vi "projekatSortiranje.vi"() -> ()   [LabVIEW 2014]
uses:
  Timer 2013/Control Timer.ctl
  Timer za drugi sprat/Control Timer2.ctl
  Timer za treci sprat/Control Timer3.ctl
  <vilib>/functionblocks/Edge Detection/Edge Detect/Edge Detect.vi
  <vilib>/functionblocks/FB Core/FB Core.xnode
  <vilib>/functionblocks/NI_FunctionBlock Libraries.lvlib
panel:
  in  "Kontrola sistema":T1(tab)
  out "Trenutno stanje":T2(ring)
  out "Trenutni paket":enum16{"Nema paketa", "P1", "P2", "P3"}(ring)
  out "Sledeci paket":enum16{"Nema paketa", "P1", "P2", "P3"}(ring)
  out "Sacuvano stanje":T2(ring)
  out "Status prvog tajmera":cluster{"Running":bool, "Done":bool}
  out "Status drugog tajmera":cluster{"Running":bool, "Done":bool}
  out "Status treceg tajmera":cluster{"Running":bool, "Done":bool}
  out "Stop":bool
  out "Emergency Stop":bool
  out "Timer Data Out za prvi sprat":T3
  out "Stanje tajmera 1 - sacuvano":enum16{"Running", "Waiting"}(ring)
  out "Stanja tajmera za sprat 1":enum16{"Running", "Waiting"}(ring)
  out "Timer Data Out za drugi sprat":T3
  out "Stanja tajmera za sprat 2":enum16{"Running", "Waiting"}(ring)
  out "Stanja tajmera 2 - sacuvano":enum16{"Running", "Waiting"}(ring)
  out "Timer Data Out za treci sprat":T3
  out "Stanja tajmera 3 - sacuvano":enum16{"Running", "Waiting"}(ring)
  out "Stanja tajmera za sprat 3":enum16{"Running", "Waiting"}(ring)
  out "Vreme 1":dbl
  out "Vreme 2":dbl
  out "Vreme 3":dbl
  in  "error in":errorcluster
  out "error out":errorcluster
  out "DO0":bool
  out "DO1":bool
  out "DO2":bool
  out "DO3":bool
  out "DO4":bool
  out "DO5":bool
  out "DO6":bool
  out "DO7":bool
  out "DO8":bool
  out "DO9":bool
  out "DO10":bool
  out "DO11":bool
  out "DO12":bool
  out "DO15":bool
  out "DO14":bool
  out "DO13":bool
  in  "Paketi":enum16{"Nema paketa", "P1", "P2", "P3"}(ring)
  in  "Stanja":T2(ring)
  in  "Stanja za odredjivanje paketa":enum16{"B2", "B4", "P3", "P2", "P1", "B3"}(ring)
  in  "Stanja tajmera za spratove":enum16{"Running", "Waiting"}(ring)
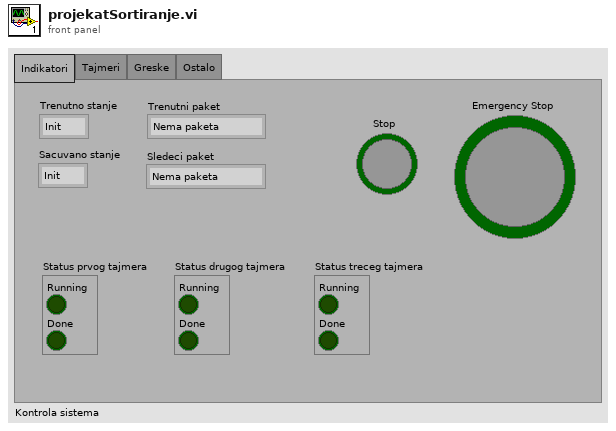
[diagram p1: front panel]
types:
  T1 = enum32{"Indikatori", "Tajmeri", "Greske", "Ostalo"}
  T2 = enum16{"Init", "Wait", "P1", "P2", "P3", "Sledeci paket", "K1", "K7", "K6", "K5", "K4", "K3", "K2", "Emergency Shutdown", "Shutdown"}
  T3 = cluster{"Last Time Stamp":dbl, "Elapsed Time":dbl}
  T4 = typedef "Control Timer3.ctl" = enum16{"Timecheck", "Reset"}
  T5 = typedef "Control Timer2.ctl" = enum16{"Timecheck", "Reset"}
  T6 = typedef "Control Timer.ctl" = enum16{"Timecheck", "Reset"}
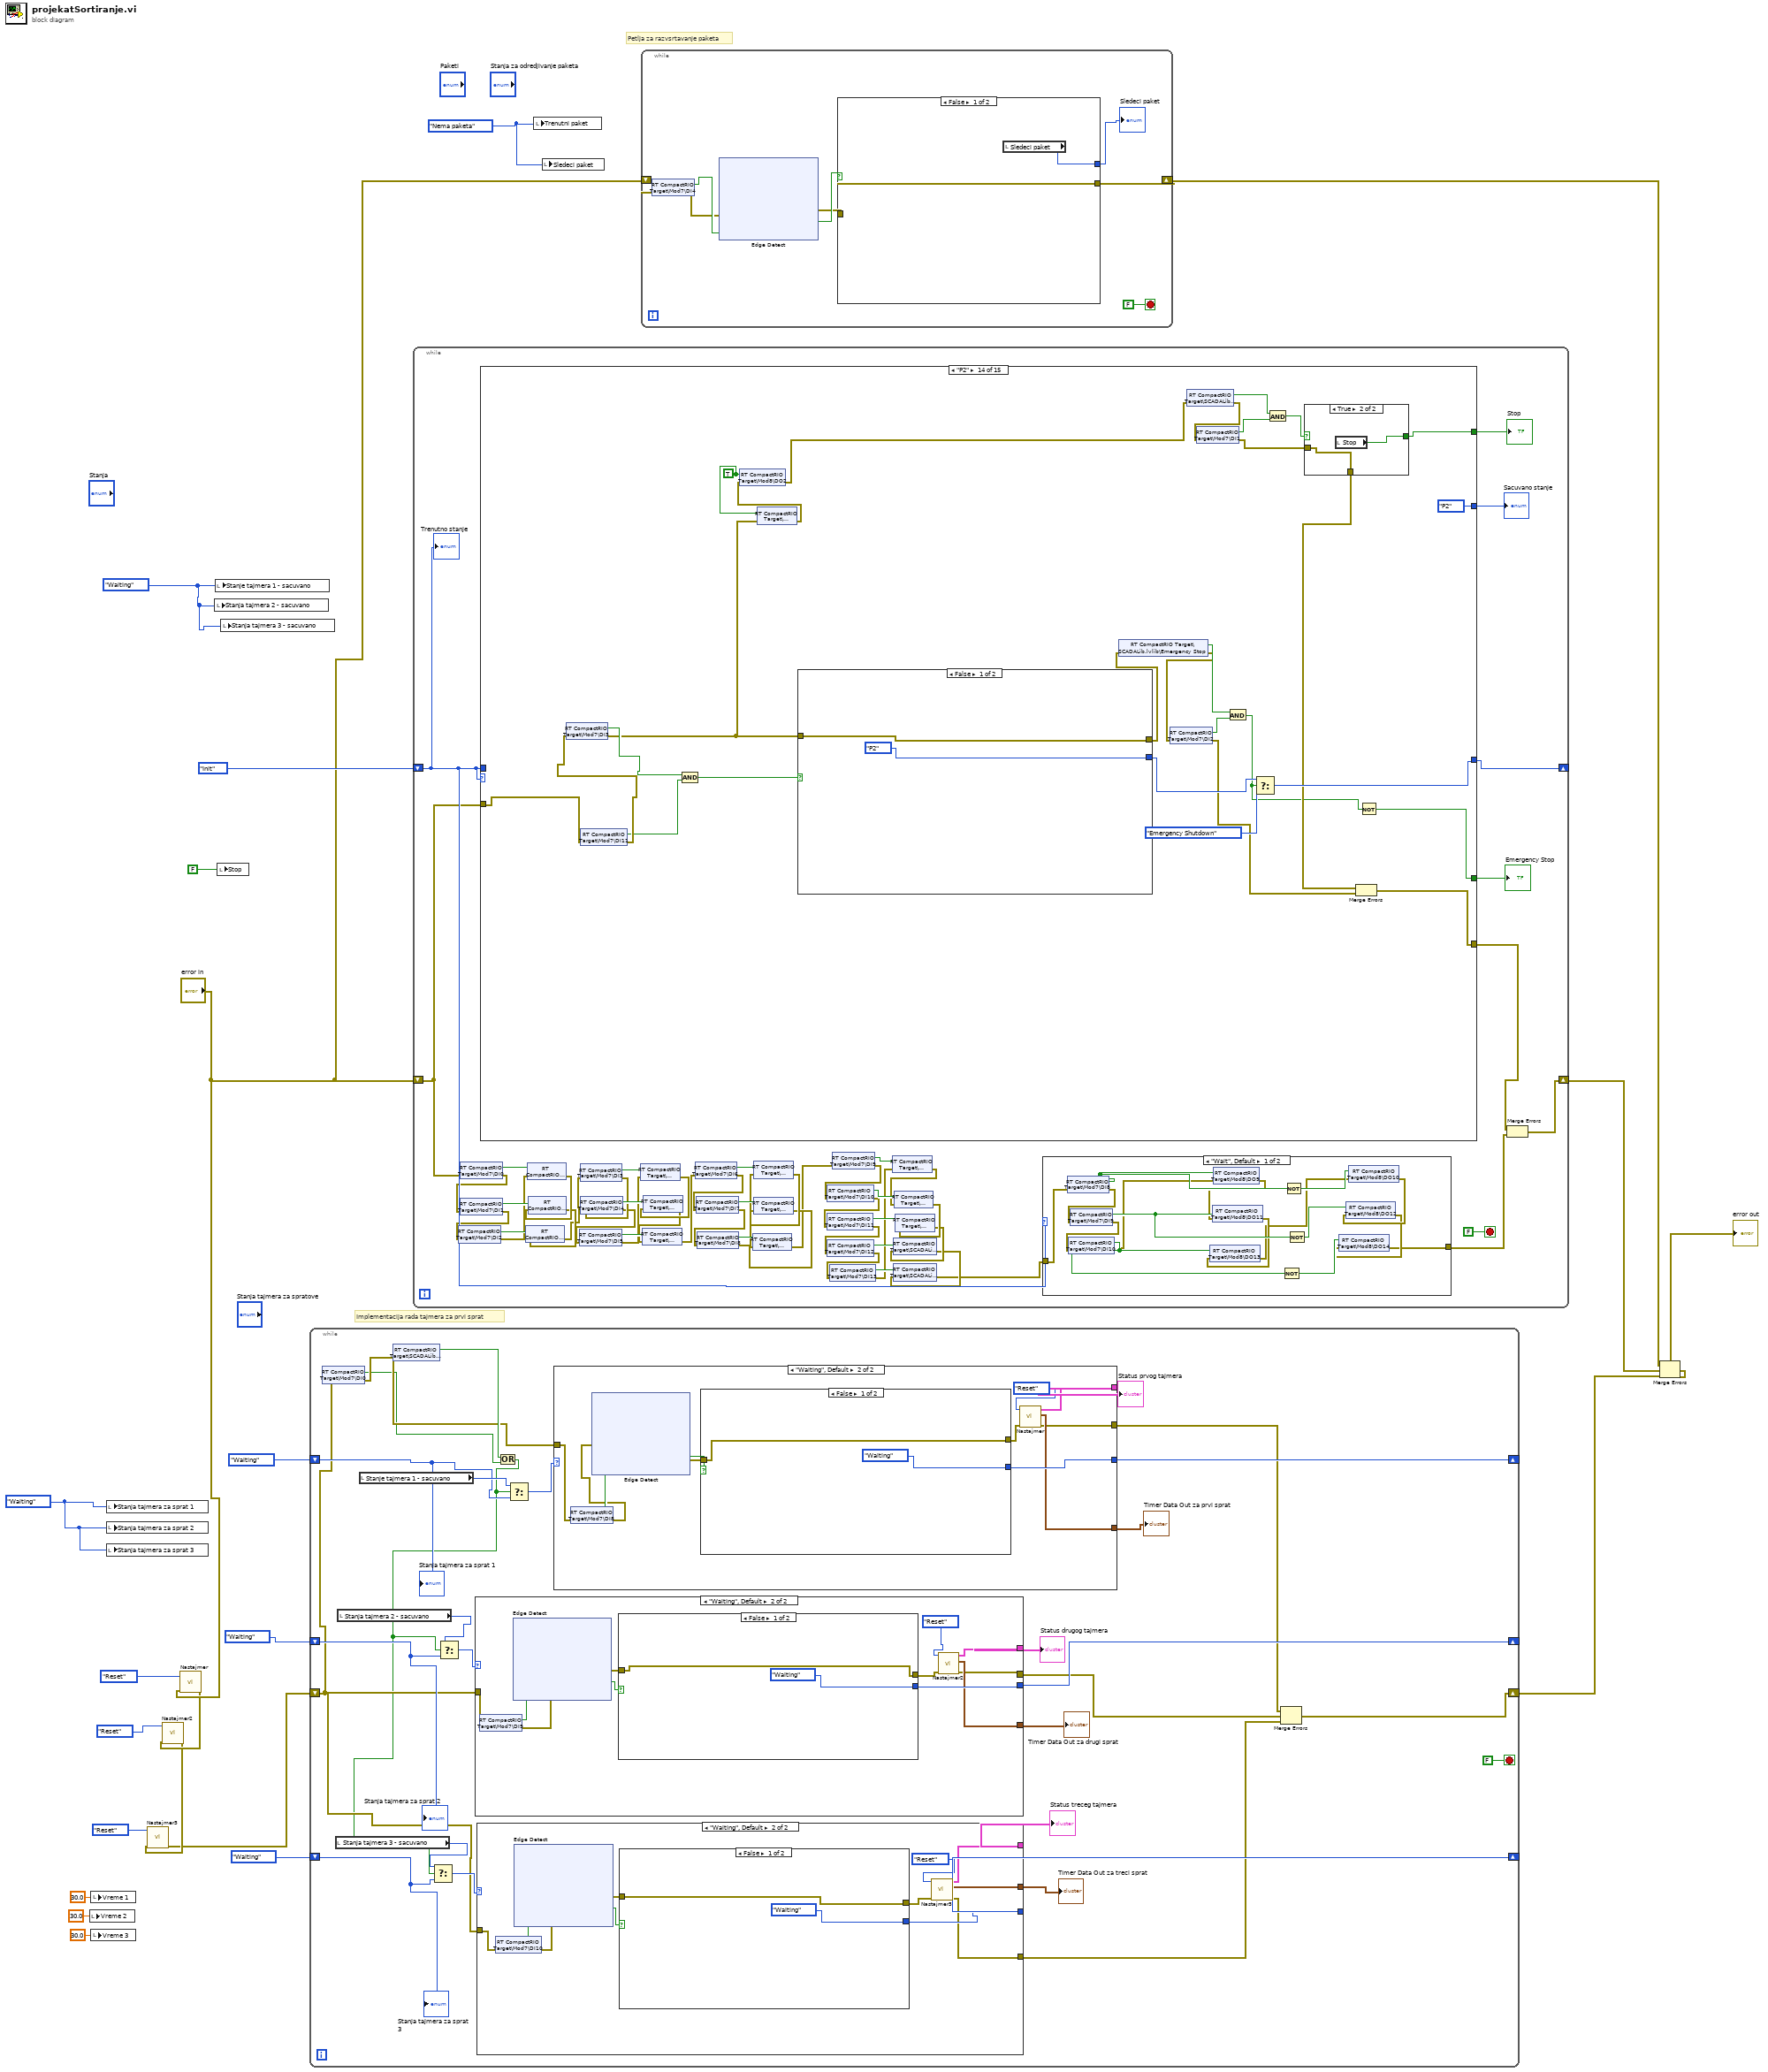
[diagram p0: block diagram]
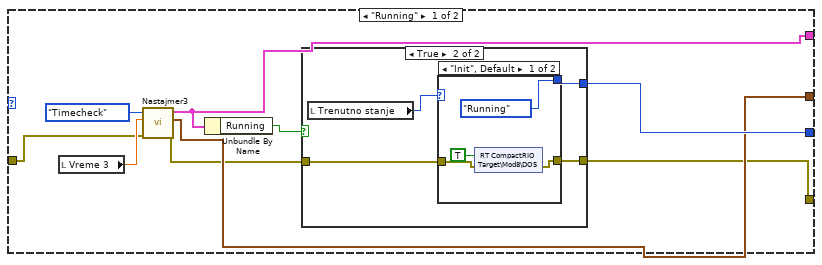
[diagram p2: hidden frame]
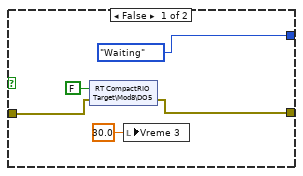
[diagram p3: hidden frame]
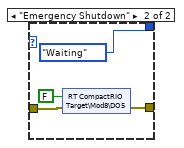
[diagram p4: hidden frame]
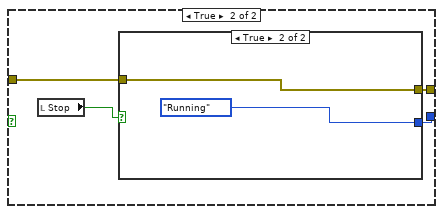
[diagram p5: hidden frame]
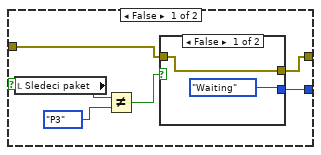
[diagram p6: hidden frame]
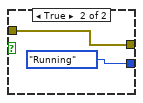
[diagram p7: hidden frame]
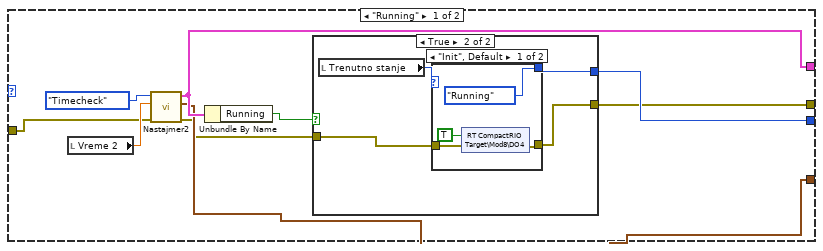
[diagram p8: hidden frame]
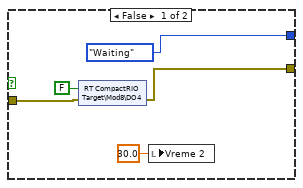
[diagram p9: hidden frame]
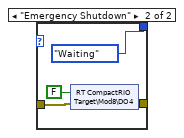
[diagram p10: hidden frame]
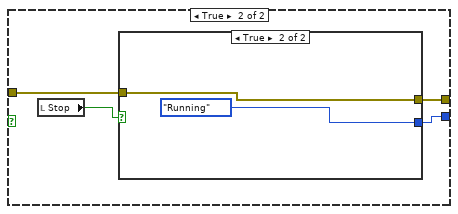
[diagram p11: hidden frame]
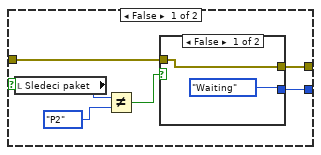
[diagram p12: hidden frame]
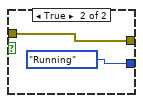
[diagram p13: hidden frame]
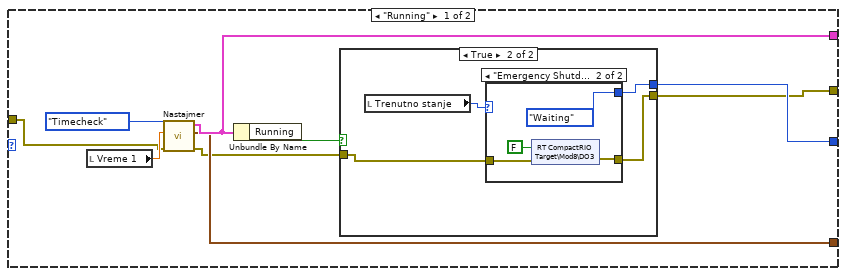
[diagram p14: hidden frame]
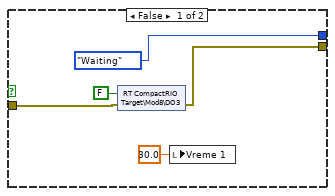
[diagram p15: hidden frame]
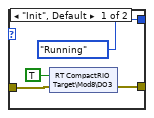
[diagram p16: hidden frame]
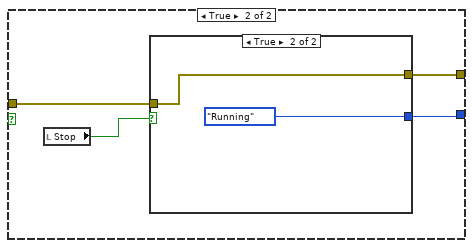
[diagram p17: hidden frame]
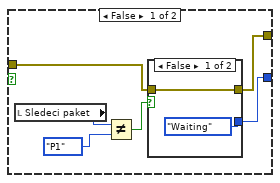
[diagram p18: hidden frame]
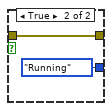
[diagram p19: hidden frame]
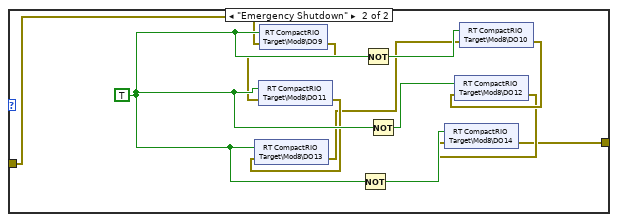
[diagram p20: hidden frame]
diagram:
  w12 = enum16{"Running", "Waiting"}."Waiting" ("Stanja tajmera za sprat 1 - sacuvano")
  w17 = enum16{"Running", "Waiting"}."Waiting" ("Stanja tajmera za spratove 1")
  w18 = enum16{"Nema paketa", "P1", "P2", "P3"}."Nema paketa" ("Trenutni paket")
  # "Implementacija rada tajmera za prvi sprat"
  # "Petlja za razvsrtavanje paketa"
  n1 = local write "Vreme 2"(30.0 ("Vreme 1")) -> ()
  n2 = local write "Vreme 1"(30.0 ("Vreme 1")) -> ()
  n3 = local write "Vreme 3"(30.0 ("Vreme 1")) -> ()
  n4 = local write "Stanja tajmera za sprat 1"(w17) -> ()
  n5 = local write "Stanja tajmera za sprat 2"(w17) -> ()
  n6 = local write "Stanja tajmera za sprat 3"(w17) -> ()
  n7 = call "Nastajmer.vi"("error in (no error)"="error in", "Enum"=Control_Timer."Reset") -> ("error out"=w4:errorcluster)  [unwired: 7 in, 2 out]
  n8 = call "Nastajmer2.vi"("error in (no error)"=w4, "Enum"=Control_Timer2."Reset") -> ("error out"=w3:errorcluster)  [unwired: 7 in, 2 out]
  n9 = call "Nastajmer3.vi"("error in (no error)"=w3, "Enum"=Control_Timer3."Reset") -> ("error out"=w2:errorcluster)  [unwired: 7 in, 2 out]
  n10 = local write "Stanja tajmera 2 - sacuvano"(w12) -> ()
  n11 = local write "Stanje tajmera 1 - sacuvano"(w12) -> ()
  n12 = local write "Stop"(FALSE ("System Stop")) -> ()
  n13 = local write "Stanja tajmera 3 - sacuvano"(w12) -> ()
  n14 = while {
    shift-right: [w49] -> _
    shift-left: enum16{"Running", "Waiting"}."Waiting" ("Stanja tajmera za spratove") -> [w40]
    shift-right: [w47] -> _
    shift-left: enum16{"Running", "Waiting"}."Waiting" ("Stanja tajmera za spratove") -> [w37]
    shift-right: [w46] -> _
    shift-left: enum16{"Running", "Waiting"}."Waiting" ("Stanja tajmera za spratove") -> [w34]
    shift-right: [w28] -> w1
    shift-left: w2 -> [w32]
    stop <- FALSE stop-if-true
    n15 = shared-variable "RT CompactRIO Target\\Mod7\\DI0"(error in=w32) -> (w23:bool, error out=w25:errorcluster)
    n16 = local read "Stanja tajmera 3 - sacuvano"() -> (w35:enum16{"Running", "Waiting"})
    n17 = local read "Stanja tajmera 2 - sacuvano"() -> (w38:enum16{"Running", "Waiting"})
    n18 = local read "Stanje tajmera 1 - sacuvano"() -> (w41:enum16{"Running", "Waiting"})
    n19 = shared-variable "RT CompactRIO Target\\SCADALib.lvlib\\Start"(error in=w25) -> (w26:bool, error out=w24:errorcluster)
    n20 = Or(x=w26, y=w23) -> (x .or. y?=w27:bool)
    n21 = Select(t=w35, s=w27, f=w34) -> (s? t:f=w33:enum16{"Running", "Waiting"})
    n22 = Select(t=w38, s=w27, f=w37) -> (s? t:f=w36:enum16{"Running", "Waiting"})
    n23 = case shown="\"Waiting\", Default" w36 {
      tunnel: [w155 w181] -> w47
      tunnel: [w153 w179] -> w48
      tunnel: [w152 w178] -> w43
      tunnel: w32 -> [w149 w177]
      tunnel: [w147 w173] -> w30
      frame "Running" {
        n24 = local read "Vreme 2"() -> (w150:dbl)
        n25 = call "Nastajmer2.vi"("error in (no error)"=w149, "Time Target"=w150, "Enum"=Control_Timer."Timecheck") -> ("error out"=w148:errorcluster, "Timer Data Out"=w152:T3, "Status"=w153:cluster{"Running":bool, "Done":bool})  [unwired: 6 in]
        n26 = Unbundle By Name(w153) -> ("Running"=w151:bool)
        n27 = case shown="True" w151 {
          tunnel: [enum16{"Running", "Waiting"}."Waiting" ("Stanja tajmera za spratove") w164] -> w155
          tunnel: w148 -> [w157 w162]
          tunnel: [w156 w161] -> w147
          frame False {
            n28 = shared-variable "RT CompactRIO Target\\Mod8\\DO4"(FALSE ("DO3"), error in=w157) -> (error out=w156:errorcluster)
            n29 = local write "Vreme 2"(30.0 ("Vreme 1")) -> ()
          }
          frame True {
            n30 = local read "Trenutno stanje"() -> (w163:T2)
            n31 = case shown="\"Init\", Default" w163 {
              tunnel: [enum16{"Running", "Waiting"}."Running" ("Stanja tajmera za spratove") enum16{"Running", "Waiting"}."Waiting" ("Stanja tajmera za spratove")] -> w164
              tunnel: w162 -> [w166 w170]
              tunnel: [w165 w169] -> w161
              frame "Init", Default {
                n32 = shared-variable "RT CompactRIO Target\\Mod8\\DO4"(TRUE ("DO3"), error in=w166) -> (error out=w165:errorcluster)
              }
              frame "Emergency Shutdown" {
                n33 = shared-variable "RT CompactRIO Target\\Mod8\\DO4"(FALSE ("DO3"), error in=w170) -> (error out=w169:errorcluster)
              }
            }
          }
        }
      }
      frame "Waiting", Default {
        n34 = shared-variable "RT CompactRIO Target\\Mod7\\DI9"(error in=w177) -> (w183:bool, error out=w176:errorcluster)
        n35 = xnode "Edge Detect"("error in"=w176, "input 2"=w183) -> ("error out"=w174:errorcluster, "output"=w182:bool)  [unwired: 1 in]
        n36 = case shown="False" w182 {
          tunnel: [enum16{"Running", "Waiting"}."Waiting" ("Stanja tajmera za spratove") w189] -> w181
          tunnel: [w184 w187] -> w175
          tunnel: w174 -> [w184 w186]
          frame False {
          }
          frame True {
            n37 = local read "Stop"() -> (w188:bool)
            n38 = case shown="True" w188 {
              tunnel: [w192 enum16{"Running", "Waiting"}."Running" ("Stanja tajmera za spratove")] -> w189
              tunnel: [w191 w200] -> w187
              tunnel: w186 -> [w190 w200]
              frame False {
                n39 = local read "Sledeci paket"() -> (w194:enum16{"Nema paketa", "P1", "P2", "P3"})
                n40 = Not Equal?(x=w194, y=enum16{"Nema paketa", "P1", "P2", "P3"}."P2" ("Paket")) -> (x != y?=w193:bool)
                n41 = case shown="False" w193 {
                  tunnel: [enum16{"Running", "Waiting"}."Waiting" ("Stanja tajmera za spratove") enum16{"Running", "Waiting"}."Running" ("Stanja tajmera za spratove")] -> w192
                  tunnel: [w196 w198] -> w191
                  tunnel: w190 -> [w196 w198]
                  frame False {
                  }
                  frame True {
                  }
                }
              }
              frame True {
              }
            }
          }
        }
        n42 = call "Nastajmer2.vi"("error in (no error)"=w175, "Enum"=Control_Timer."Reset") -> ("error out"=w173:errorcluster, "Timer Data Out"=w178:T3, "Status"=w179:cluster{"Running":bool, "Done":bool})  [unwired: 7 in]
      }
    }
    "Status drugog tajmera" <- w48
    "Timer Data Out za drugi sprat" <- w43
    n43 = case shown="\"Waiting\", Default" w33 {
      tunnel: [w60 w86] -> w46
      tunnel: [w57 w84] -> w45
      tunnel: [w58 w83] -> w42
      tunnel: w32 -> [w54 w82]
      tunnel: [w52 w78] -> w31
      frame "Running" {
        n44 = local read "Vreme 3"() -> (w55:dbl)
        n45 = call "Nastajmer3.vi"("error in (no error)"=w54, "Time Target"=w55, "Enum"=Control_Timer."Timecheck") -> ("error out"=w53:errorcluster, "Timer Data Out"=w58:T3, "Status"=w57:cluster{"Running":bool, "Done":bool})  [unwired: 6 in]
        n46 = Unbundle By Name(w57) -> ("Running"=w56:bool)
        n47 = case shown="True" w56 {
          tunnel: [enum16{"Running", "Waiting"}."Waiting" ("Stanja tajmera za spratove") w69] -> w60
          tunnel: w53 -> [w62 w67]
          tunnel: [w61 w66] -> w52
          frame False {
            n48 = shared-variable "RT CompactRIO Target\\Mod8\\DO5"(FALSE ("DO3"), error in=w62) -> (error out=w61:errorcluster)
            n49 = local write "Vreme 3"(30.0 ("Vreme 1")) -> ()
          }
          frame True {
            n50 = local read "Trenutno stanje"() -> (w68:T2)
            n51 = case shown="\"Init\", Default" w68 {
              tunnel: [enum16{"Running", "Waiting"}."Running" ("Stanja tajmera za spratove") enum16{"Running", "Waiting"}."Waiting" ("Stanja tajmera za spratove")] -> w69
              tunnel: w67 -> [w71 w75]
              tunnel: [w70 w74] -> w66
              frame "Init", Default {
                n52 = shared-variable "RT CompactRIO Target\\Mod8\\DO5"(TRUE ("DO3"), error in=w71) -> (error out=w70:errorcluster)
              }
              frame "Emergency Shutdown" {
                n53 = shared-variable "RT CompactRIO Target\\Mod8\\DO5"(FALSE ("DO3"), error in=w75) -> (error out=w74:errorcluster)
              }
            }
          }
        }
      }
      frame "Waiting", Default {
        n54 = shared-variable "RT CompactRIO Target\\Mod7\\DI10"(error in=w82) -> (w88:bool, error out=w81:errorcluster)
        n55 = xnode "Edge Detect"("error in"=w81, "input 2"=w88) -> ("error out"=w80:errorcluster, "output"=w87:bool)  [unwired: 1 in]
        n56 = case shown="False" w87 {
          tunnel: [enum16{"Running", "Waiting"}."Waiting" ("Stanja tajmera za spratove") w94] -> w86
          tunnel: [w89 w92] -> w79
          tunnel: w80 -> [w89 w91]
          frame False {
          }
          frame True {
            n57 = local read "Stop"() -> (w93:bool)
            n58 = case shown="True" w93 {
              tunnel: [w97 enum16{"Running", "Waiting"}."Running" ("Stanja tajmera za spratove")] -> w94
              tunnel: [w96 w105] -> w92
              tunnel: w91 -> [w95 w105]
              frame False {
                n59 = local read "Sledeci paket"() -> (w99:enum16{"Nema paketa", "P1", "P2", "P3"})
                n60 = Not Equal?(x=w99, y=enum16{"Nema paketa", "P1", "P2", "P3"}."P3" ("Paket")) -> (x != y?=w98:bool)
                n61 = case shown="False" w98 {
                  tunnel: [enum16{"Running", "Waiting"}."Waiting" ("Stanja tajmera za spratove") enum16{"Running", "Waiting"}."Running" ("Stanja tajmera za spratove")] -> w97
                  tunnel: [w101 w103] -> w96
                  tunnel: w95 -> [w101 w103]
                  frame False {
                  }
                  frame True {
                  }
                }
              }
              frame True {
              }
            }
          }
        }
        n62 = call "Nastajmer3.vi"("error in (no error)"=w79, "Enum"=Control_Timer."Reset") -> ("error out"=w78:errorcluster, "Timer Data Out"=w83:T3, "Status"=w84:cluster{"Running":bool, "Done":bool})  [unwired: 7 in]
      }
    }
    "Status treceg tajmera" <- w45
    "Timer Data Out za treci sprat" <- w42
    n63 = Select(t=w41, s=w27, f=w40) -> (s? t:f=w39:enum16{"Running", "Waiting"})
    n64 = case shown="\"Waiting\", Default" w39 {
      tunnel: [w250 w277] -> w49
      tunnel: [w247 w274] -> w50
      tunnel: [w246 w273] -> w44
      tunnel: w24 -> [w244 w272]
      tunnel: [w242 w268] -> w29
      frame "Running" {
        n65 = local read "Vreme 1"() -> (w245:dbl)
        n66 = call "Nastajmer.vi"("error in (no error)"=w244, "Time Target"=w245, "Enum"=Control_Timer."Timecheck") -> ("error out"=w243:errorcluster, "Timer Data Out"=w246:T3, "Status"=w247:cluster{"Running":bool, "Done":bool})  [unwired: 6 in]
        n67 = Unbundle By Name(w247) -> ("Running"=w248:bool)
        n68 = case shown="True" w248 {
          tunnel: [enum16{"Running", "Waiting"}."Waiting" ("Stanja tajmera za spratove") w259] -> w250
          tunnel: w243 -> [w252 w257]
          tunnel: [w251 w256] -> w242
          frame False {
            n69 = shared-variable "RT CompactRIO Target\\Mod8\\DO3"(FALSE ("DO3"), error in=w252) -> (error out=w251:errorcluster)
            n70 = local write "Vreme 1"(30.0 ("Vreme 1")) -> ()
          }
          frame True {
            n71 = local read "Trenutno stanje"() -> (w258:T2)
            n72 = case shown="\"Emergency Shutdown\"" w258 {
              tunnel: [enum16{"Running", "Waiting"}."Running" ("Stanja tajmera za spratove") enum16{"Running", "Waiting"}."Waiting" ("Stanja tajmera za spratove")] -> w259
              tunnel: w257 -> [w261 w265]
              tunnel: [w260 w264] -> w256
              frame "Init", Default {
                n73 = shared-variable "RT CompactRIO Target\\Mod8\\DO3"(TRUE ("DO3"), error in=w261) -> (error out=w260:errorcluster)
              }
              frame "Emergency Shutdown" {
                n74 = shared-variable "RT CompactRIO Target\\Mod8\\DO3"(FALSE ("DO3"), error in=w265) -> (error out=w264:errorcluster)
              }
            }
          }
        }
      }
      frame "Waiting", Default {
        n75 = shared-variable "RT CompactRIO Target\\Mod7\\DI8"(error in=w272) -> (w278:bool, error out=w271:errorcluster)
        n76 = xnode "Edge Detect"("error in"=w271, "input 2"=w278) -> ("error out"=w269:errorcluster, "output"=w276:bool)  [unwired: 1 in]
        n77 = case shown="False" w276 {
          tunnel: [enum16{"Running", "Waiting"}."Waiting" ("Stanja tajmera za spratove") w283] -> w277
          tunnel: [w279 w282] -> w270
          tunnel: w269 -> [w279 w281]
          frame False {
          }
          frame True {
            n78 = local read "Stop"() -> (w284:bool)
            n79 = case shown="True" w284 {
              tunnel: [w287 enum16{"Running", "Waiting"}."Running" ("Stanja tajmera za spratove")] -> w283
              tunnel: [w286 w295] -> w282
              tunnel: w281 -> [w285 w295]
              frame False {
                n80 = local read "Sledeci paket"() -> (w290:enum16{"Nema paketa", "P1", "P2", "P3"})
                n81 = Not Equal?(x=w290, y=enum16{"Nema paketa", "P1", "P2", "P3"}."P1" ("Paket")) -> (x != y?=w288:bool)
                n82 = case shown="False" w288 {
                  tunnel: [enum16{"Running", "Waiting"}."Waiting" ("Stanja tajmera za spratove") enum16{"Running", "Waiting"}."Running" ("Stanja tajmera za spratove")] -> w287
                  tunnel: [w291 w293] -> w286
                  tunnel: w285 -> [w291 w293]
                  frame False {
                  }
                  frame True {
                  }
                }
              }
              frame True {
              }
            }
          }
        }
        n83 = call "Nastajmer.vi"("error in (no error)"=w270, "Enum"=Control_Timer."Reset") -> ("error out"=w268:errorcluster, "Timer Data Out"=w273:T3, "Status"=w274:cluster{"Running":bool, "Done":bool})  [unwired: 7 in]
      }
    }
    "Status prvog tajmera" <- w50
    "Timer Data Out za prvi sprat" <- w44
    n84 = Merge Errors(w29, w30, w31) -> (w28:errorcluster)
    "Stanja tajmera za sprat 1" <- w40
    "Stanja tajmera za sprat 2" <- w37
    "Stanja tajmera za sprat 3" <- w34
  }
  n85 = while {
    shift-right: [w380] -> w7
    shift-left: "error in" -> [w365]
    shift-right: [w387] -> _
    shift-left: T2."Init" ("Stanja") -> [w383]
    stop <- FALSE stop-if-true
    n86 = shared-variable "RT CompactRIO Target\\Mod7\\DI0"(error in=w365) -> (w379:bool, error out=w364:errorcluster)
    n87 = shared-variable "RT CompactRIO Target\\Mod7\\DI1"(error in=w364) -> (w378:bool, error out=w363:errorcluster)
    n88 = shared-variable "RT CompactRIO Target\\Mod7\\DI2"(error in=w363) -> (w377:bool, error out=w362:errorcluster)
    n89 = case shown="\"P2\"" w383 {
      tunnel: [w416 w467 w506 w545 w631 w791 w860 w957 w990 w1034 w1066 w1229 w1253 w1292 w1331] -> w381
      tunnel: [w446 w474 w505 w566 w633 w788 w859 w968 w1003 w1038 w1073 w1233 w1264 w1303 w1342] -> w387
      tunnel: w383 -> [_ _ _ _ _ _ _ _ _ _ _ w1233 _ _ _]
      tunnel: w365 -> [w418 w453 w482 w550 w629 w800 w851 w965 w1000 w1023 w1054 w1224 w1261 w1300 w1339]
      tunnel: [w447 w473 w501 w562 w618 w803 w847 w961 w996 w1030 w1074 w1232 w1258 w1297 w1336] -> w386
      tunnel: [w444 w470 w498 w559 w616 w802 w845 w959 w994 w1028 w1058 FALSE w1256 w1294 w1334] -> w385
      tunnel: [T2."Init" ("Stanja") T2."Wait" ("Stanja") T2."K1" ("Stanja") T2."Sledeci paket" ("Stanja") T2."K7" ("Stanja") T2."K6" ("Stanja") T2."K5" ("Stanja") T2."K3" ("Stanja") T2."K4" ("Stanja") T2."K2" ("Stanja") w1072 T2."Shutdown" ("Sacuvano stanje") T2."P1" ("Sacuvano stanje") T2."P2" ("Sacuvano stanje") T2."P3" ("Sacuvano stanje")] -> w384
      frame "Init" {
        w434 = FALSE
        n90 = shared-variable "RT CompactRIO Target\\Mod8\\DO0"(w434, error in=w418) -> (error out=w433:errorcluster)
        n91 = shared-variable "RT CompactRIO Target\\Mod8\\DO1"(w434, error in=w433) -> (error out=w432:errorcluster)
        n92 = shared-variable "RT CompactRIO Target\\Mod8\\DO2"(w434, error in=w432) -> (error out=w431:errorcluster)
        n93 = shared-variable "RT CompactRIO Target\\Mod8\\DO3"(w434, error in=w431) -> (error out=w430:errorcluster)
        n94 = shared-variable "RT CompactRIO Target\\Mod8\\DO4"(w434, error in=w430) -> (error out=w429:errorcluster)
        n95 = shared-variable "RT CompactRIO Target\\Mod8\\DO5"(w434, error in=w429) -> (error out=w428:errorcluster)
        n96 = shared-variable "RT CompactRIO Target\\Mod8\\DO6"(w434, error in=w428) -> (error out=w427:errorcluster)
        n97 = shared-variable "RT CompactRIO Target\\Mod8\\DO7"(w434, error in=w427) -> (error out=w424:errorcluster)
        n98 = shared-variable "RT CompactRIO Target\\Mod8\\DO8"(w434, error in=w424) -> (error out=w426:errorcluster)
        n99 = shared-variable "RT CompactRIO Target\\Mod8\\DO9"(w434, error in=w426) -> (error out=w423:errorcluster)
        n100 = shared-variable "RT CompactRIO Target\\Mod8\\DO10"(w434, error in=w423) -> (error out=w425:errorcluster)
        n101 = shared-variable "RT CompactRIO Target\\Mod8\\DO11"(w434, error in=w425) -> (error out=w422:errorcluster)
        n102 = shared-variable "RT CompactRIO Target\\Mod8\\DO12"(w434, error in=w422) -> (error out=w421:errorcluster)
        n103 = shared-variable "RT CompactRIO Target\\Mod8\\DO13"(w434, error in=w421) -> (error out=w420:errorcluster)
        n104 = shared-variable "RT CompactRIO Target\\Mod8\\DO14"(w434, error in=w420) -> (error out=w419:errorcluster)
        n105 = shared-variable "RT CompactRIO Target\\Mod8\\DO15"(w434, error in=w419) -> (error out=w417:errorcluster)
        n106 = shared-variable "RT CompactRIO Target\\SCADALib.lvlib\\Stop"(error in=w417) -> (w439:bool, error out=w441:errorcluster)
        n107 = shared-variable "RT CompactRIO Target\\Mod7\\DI1"(error in=w441) -> (w438:bool, error out=w440:errorcluster)
        n108 = And(x=w439, y=w438) -> (x .and. y?=w442:bool)
        n109 = case shown="True" w442 {
          tunnel: [TRUE w451] -> w447
          tunnel: w440 -> [w448 w450]
          tunnel: [w448 w450] -> w437
          frame False {
          }
          frame True {
            n110 = local read "Stop"() -> (w451:bool)
          }
        }
        n111 = shared-variable "RT CompactRIO Target\\Mod7\\DI2"(error in=w437) -> (w445:bool, error out=w416:errorcluster)
        n112 = Not(x=w445) -> (.not. x?=w444:bool)
        n113 = Select(t=T2."Wait" ("Stanja"), s=w445, f=T2."Emergency Shutdown" ("Stanja")) -> (s? t:f=w446:T2)
      }
      frame "Wait" {
        n114 = shared-variable "RT CompactRIO Target\\SCADALib.lvlib\\Start"(error in=w453) -> (w464:bool, error out=w452:errorcluster)
        n115 = shared-variable "RT CompactRIO Target\\Mod7\\DI0"(error in=w452) -> (w466:bool, error out=w455:errorcluster)
        n116 = Or(x=w466, y=w464) -> (x .or. y?=w465:bool)
        n117 = Select(t=T2."K1" ("Stanja"), s=w465, f=T2."Wait" ("Stanja")) -> (s? t:f=w472:T2)
        n118 = shared-variable "RT CompactRIO Target\\SCADALib.lvlib\\Emergency Stop"(error in=w455) -> (w461:bool, error out=w454:errorcluster)
        n119 = shared-variable "RT CompactRIO Target\\Mod7\\DI2"(error in=w454) -> (w462:bool, error out=w457:errorcluster)
        n120 = And(x=w462, y=w461) -> (x .and. y?=w463:bool)
        n121 = Select(t=w472, s=w463, f=T2."Emergency Shutdown" ("Stanja")) -> (s? t:f=w474:T2)
        n122 = Not(x=w463) -> (.not. x?=w470:bool)
        n123 = shared-variable "RT CompactRIO Target\\SCADALib.lvlib\\Stop"(error in=w457) -> (w458:bool, error out=w456:errorcluster)
        n124 = shared-variable "RT CompactRIO Target\\Mod7\\DI1"(error in=w456) -> (w460:bool, error out=w468:errorcluster)
        n125 = And(x=w458, y=w460) -> (x .and. y?=w459:bool)
        n126 = case shown="True" w459 {
          tunnel: [TRUE w480] -> w473
          tunnel: [w477 w479] -> w467
          tunnel: w468 -> [w477 w479]
          frame False {
          }
          frame True {
            n127 = local read "Stop"() -> (w480:bool)
          }
        }
      }
      frame "K1" {
        w483 = TRUE ("K1")
        n128 = local read "Sledeci paket"() -> (w504:enum16{"Nema paketa", "P1", "P2", "P3"})
        n129 = shared-variable "RT CompactRIO Target\\SCADALib.lvlib\\On-Off"(w483, error in=w482) -> (error out=w481:errorcluster)
        n130 = shared-variable "RT CompactRIO Target\\Mod8\\DO0"(w483, error in=w481) -> (error out=w491:errorcluster)
        n131 = shared-variable "RT CompactRIO Target\\SCADALib.lvlib\\Emergency Stop"(error in=w491) -> (w492:bool, error out=w490:errorcluster)
        n132 = shared-variable "RT CompactRIO Target\\Mod7\\DI2"(error in=w490) -> (w493:bool, error out=w485:errorcluster)
        n133 = And(x=w492, y=w493) -> (x .and. y?=w494:bool)
        n134 = case shown="\"Nema paketa\"" w504 {
          tunnel: [T2."K1" ("Stanja") T2."Sledeci paket" ("Stanja")] -> w500
          tunnel: [w512 w514] -> w495
          tunnel: w482 -> [w512 w514]
          frame "Nema paketa" {
          }
          frame "P1", Default {
          }
        }
        n135 = shared-variable "RT CompactRIO Target\\Mod7\\DI3"(error in=w495) -> (w502:bool, error out=w503:errorcluster)
        n136 = Select(t=w500, s=w494, f=T2."Emergency Shutdown" ("Stanja")) -> (s? t:f=w505:T2)
        n137 = case shown="False" w502 {
          tunnel: w503 -> [w517 w522]
          tunnel: [w519 w523] -> w507
          frame False {
            w518 = TRUE ("K1")
            n138 = shared-variable "RT CompactRIO Target\\SCADALib.lvlib\\K1"(w518, error in=w517) -> (error out=w516:errorcluster)
            n139 = shared-variable "RT CompactRIO Target\\Mod8\\DO2"(w518, error in=w516) -> (error out=w519:errorcluster)
          }
          frame True {
            n140 = shared-variable "RT CompactRIO Target\\Mod7\\DI11"(error in=w522) -> (w521:bool, error out=w520:errorcluster)
            n141 = case shown="False" w521 {
              tunnel: w520 -> [w525 w529]
              tunnel: [w527 w531] -> w523
              frame False {
                w526 = FALSE ("K1")
                n142 = shared-variable "RT CompactRIO Target\\SCADALib.lvlib\\K1"(w526, error in=w525) -> (error out=w524:errorcluster)
                n143 = shared-variable "RT CompactRIO Target\\Mod8\\DO2"(w526, error in=w524) -> (error out=w527:errorcluster)
              }
              frame True {
                n144 = shared-variable "RT CompactRIO Target\\Mod7\\DI7"(error in=w529) -> (w530:bool, error out=w528:errorcluster)
                n145 = case shown="True" w530 {
                  tunnel: w528 -> [w533 w537]
                  tunnel: [w535 w539] -> w531
                  frame False {
                    w534 = TRUE ("K1")
                    n146 = shared-variable "RT CompactRIO Target\\SCADALib.lvlib\\K1"(w534, error in=w533) -> (error out=w532:errorcluster)
                    n147 = shared-variable "RT CompactRIO Target\\Mod8\\DO2"(w534, error in=w532) -> (error out=w535:errorcluster)
                  }
                  frame True {
                    w538 = FALSE ("K1")
                    n148 = shared-variable "RT CompactRIO Target\\SCADALib.lvlib\\K1"(w538, error in=w537) -> (error out=w536:errorcluster)
                    n149 = shared-variable "RT CompactRIO Target\\Mod8\\DO2"(w538, error in=w536) -> (error out=w539:errorcluster)
                  }
                }
              }
            }
          }
        }
        n150 = Not(x=w494) -> (.not. x?=w498:bool)
        n151 = shared-variable "RT CompactRIO Target\\Mod7\\DI1"(error in=w485) -> (w489:bool, error out=w486:errorcluster)
        n152 = shared-variable "RT CompactRIO Target\\SCADALib.lvlib\\Stop"(error in=w486) -> (w487:bool, error out=w484:errorcluster)
        n153 = And(x=w487, y=w489) -> (x .and. y?=w488:bool)
        n154 = case shown="False" w488 {
          tunnel: [TRUE w511] -> w501
          tunnel: [w508 w510] -> w496
          tunnel: w484 -> [w508 w510]
          frame False {
          }
          frame True {
            n155 = local read "Stop"() -> (w511:bool)
          }
        }
        n156 = Merge Errors(w496, w507) -> (w506:errorcluster)
      }
      frame "Sledeci paket" {
        w543 = FALSE ("K6")
        n157 = shared-variable "RT CompactRIO Target\\Mod8\\DO8"(FALSE ("K7"), error in=w550) -> (error out=w557:errorcluster)
        n158 = local read "Stop"() -> (w563:bool)
        n159 = shared-variable "RT CompactRIO Target\\Mod8\\DO7"(w543, error in=w557) -> (error out=w542:errorcluster)
        n160 = shared-variable "RT CompactRIO Target\\SCADALib.lvlib\\K6"(w543, error in=w542) -> (error out=w541:errorcluster)
        n161 = shared-variable "RT CompactRIO Target\\SCADALib.lvlib\\K7"(w543, error in=w541) -> (error out=w540:errorcluster)
        n162 = case shown="True" w563 {
          tunnel: [T2."Sledeci paket" ("Stanja") w588] -> w561
          tunnel: [enum16{"Nema paketa", "P1", "P2", "P3"}."Nema paketa" ("Paketi") w586] -> w565
          tunnel: [w575 w584] -> w549
          tunnel: w540 -> [w573 w583]
          frame True {
            w574 = FALSE ("DO2")
            n163 = shared-variable "RT CompactRIO Target\\Mod8\\DO2"(w574, error in=w573) -> (error out=w572:errorcluster)
            n164 = shared-variable "RT CompactRIO Target\\SCADALib.lvlib\\K1"(w574, error in=w572) -> (error out=w571:errorcluster)
            n165 = shared-variable "RT CompactRIO Target\\Mod8\\DO6"(w574, error in=w571) -> (error out=w576:errorcluster)
            n166 = shared-variable "RT CompactRIO Target\\Mod8\\DO0"(w574, error in=w576) -> (error out=w575:errorcluster)
          }
          frame False {
            w581 = TRUE ("DO2")
            n167 = local read "Sledeci paket"() -> (w587:enum16{"Nema paketa", "P1", "P2", "P3"})
            n168 = shared-variable "RT CompactRIO Target\\SCADALib.lvlib\\On-Off"(w581, error in=w583) -> (error out=w582:errorcluster)
            n169 = shared-variable "RT CompactRIO Target\\Mod8\\DO0"(w581, error in=w582) -> (error out=w585:errorcluster)
            n170 = shared-variable "RT CompactRIO Target\\Mod8\\DO2"(w581, error in=w585) -> (error out=w580:errorcluster)
            n171 = shared-variable "RT CompactRIO Target\\SCADALib.lvlib\\K1"(w581, error in=w580) -> (error out=w579:errorcluster)
            n172 = case shown="\"P1\"" w587 {
              tunnel: [T2."Sledeci paket" ("Stanja") T2."P1" ("Stanja") T2."P2" ("Stanja") T2."P3" ("Stanja")] -> w588
              tunnel: [enum16{"Nema paketa", "P1", "P2", "P3"}."Nema paketa" ("Paketi") enum16{"Nema paketa", "P1", "P2", "P3"}."P1" ("Paketi") enum16{"Nema paketa", "P1", "P2", "P3"}."P2" ("Paketi") enum16{"Nema paketa", "P1", "P2", "P3"}."P3" ("Paketi")] -> w586
              tunnel: [w589 w592 w595 w598] -> w584
              tunnel: w579 -> [w589 w592 w595 w598]
              frame "Nema paketa", Default {
              }
              frame "P1" {
              }
              frame "P2" {
              }
              frame "P3" {
              }
            }
          }
        }
        "Trenutni paket" <- w565
        n173 = shared-variable "RT CompactRIO Target\\SCADALib.lvlib\\Emergency Stop"(error in=w549) -> (w544:bool, error out=w548:errorcluster)
        n174 = shared-variable "RT CompactRIO Target\\Mod7\\DI2"(error in=w548) -> (w555:bool, error out=w547:errorcluster)
        n175 = shared-variable "RT CompactRIO Target\\SCADALib.lvlib\\Start"(error in=w547) -> (w552:bool, error out=w546:errorcluster)
        n176 = shared-variable "RT CompactRIO Target\\Mod7\\DI0"(error in=w546) -> (w554:bool, error out=w556:errorcluster)
        n177 = Or(x=w552, y=w554) -> (x .or. y?=w553:bool)
        n178 = case shown="True" w553 {
          tunnel: [w568 FALSE] -> w562
          tunnel: [w567 w569] -> w545
          tunnel: w556 -> [w567 w569]
          frame False {
            n179 = local read "Stop"() -> (w568:bool)
          }
          frame True {
          }
        }
        n180 = And(x=w544, y=w555) -> (x .and. y?=w551:bool)
        n181 = Select(t=w561, s=w551, f=T2."Emergency Shutdown" ("Stanja")) -> (s? t:f=w566:T2)
        n182 = Not(x=w551) -> (.not. x?=w559:bool)
      }
      frame "K7" {
        n183 = shared-variable "RT CompactRIO Target\\Mod7\\DI3"(error in=w629) -> (w620:bool, error out=w626:errorcluster)
        n184 = shared-variable "RT CompactRIO Target\\Mod7\\DI3"(error in=w629) -> (w627:bool, error out=w628:errorcluster)
        n185 = shared-variable "RT CompactRIO Target\\Mod7\\DI7"(error in=w626) -> (w625:bool, error out=w621:errorcluster)
        n186 = shared-variable "RT CompactRIO Target\\Mod7\\DI7"(error in=w621) -> (w624:bool, error out=w623:errorcluster)
        n187 = Not(x=w624) -> (.not. x?=w603:bool)
        n188 = Not(x=w620) -> (.not. x?=w619:bool)
        n189 = Or(x=w619, y=w625) -> (x .or. y?=w634:bool)
        n190 = shared-variable "RT CompactRIO Target\\Mod8\\DO6"(w603, error in=w623) -> (error out=w602:errorcluster)
        n191 = shared-variable "RT CompactRIO Target\\SCADALib.lvlib\\K5"(w603, error in=w602) -> (error out=w601:errorcluster)
        n192 = case shown="True" w634 {
          tunnel: [w645 T2."K7" ("Stanja")] -> w630
          tunnel: w601 -> [w642 w757]
          tunnel: [w644 w754] -> w622
          frame True {
            w641 = TRUE ("K7")
            n193 = local read "Trenutni paket"() -> (w643:enum16{"Nema paketa", "P1", "P2", "P3"})
            n194 = shared-variable "RT CompactRIO Target\\Mod8\\DO8"(w641, error in=w642) -> (error out=w640:errorcluster)
            n195 = shared-variable "RT CompactRIO Target\\SCADALib.lvlib\\K7"(w641, error in=w640) -> (error out=w639:errorcluster)
            n196 = case shown="\"P3\"" w643 {
              tunnel: [w651 w705] -> w645
              tunnel: w639 -> [w650 w704]
              tunnel: [w646 w700] -> w644
              frame "P2", Default {
                n197 = shared-variable "RT CompactRIO Target\\Mod7\\DI12"(error in=w650) -> (w648:bool, error out=w649:errorcluster)
                n198 = xnode "Edge Detect"("error in"=w649, "input 1"=w648) -> ("error out"=w647:errorcluster, "output"=w652:bool)  [unwired: 1 in]
                n199 = case shown="True" w652 {
                  tunnel: [T2."K7" ("Stanja") T2."K3" ("Stanja")] -> w651
                  tunnel: w647 -> [w693 w698]
                  tunnel: [w693 w695] -> w646
                  frame False {
                  }
                  frame True {
                    w697 = FALSE ("K7")
                    n200 = shared-variable "RT CompactRIO Target\\Mod8\\DO8"(w697, error in=w698) -> (error out=w696:errorcluster)
                    n201 = shared-variable "RT CompactRIO Target\\SCADALib.lvlib\\K7"(w697, error in=w696) -> (error out=w695:errorcluster)
                  }
                }
              }
              frame "P3" {
                n202 = shared-variable "RT CompactRIO Target\\Mod7\\DI13"(error in=w704) -> (w702:bool, error out=w703:errorcluster)
                n203 = xnode "Edge Detect"("error in"=w703, "input 1"=w702) -> ("error out"=w701:errorcluster, "output"=w706:bool)  [unwired: 1 in]
                n204 = case shown="True" w706 {
                  tunnel: [T2."K7" ("Stanja") T2."K4" ("Stanja")] -> w705
                  tunnel: w701 -> [w747 w752]
                  tunnel: [w747 w749] -> w700
                  frame False {
                  }
                  frame True {
                    w751 = FALSE ("K7")
                    n205 = shared-variable "RT CompactRIO Target\\Mod8\\DO8"(w751, error in=w752) -> (error out=w750:errorcluster)
                    n206 = shared-variable "RT CompactRIO Target\\SCADALib.lvlib\\K7"(w751, error in=w750) -> (error out=w749:errorcluster)
                  }
                }
              }
            }
          }
          frame False {
            w756 = FALSE ("K7")
            n207 = shared-variable "RT CompactRIO Target\\Mod8\\DO8"(w756, error in=w757) -> (error out=w755:errorcluster)
            n208 = shared-variable "RT CompactRIO Target\\SCADALib.lvlib\\K7"(w756, error in=w755) -> (error out=w754:errorcluster)
          }
        }
        n209 = case shown="True" w627 {
          tunnel: w628 -> [w760 w765]
          tunnel: [w762 w766] -> w632
          frame False {
            w761 = TRUE ("K1")
            n210 = shared-variable "RT CompactRIO Target\\SCADALib.lvlib\\K1"(w761, error in=w760) -> (error out=w759:errorcluster)
            n211 = shared-variable "RT CompactRIO Target\\Mod8\\DO2"(w761, error in=w759) -> (error out=w762:errorcluster)
          }
          frame True {
            n212 = shared-variable "RT CompactRIO Target\\Mod7\\DI11"(error in=w765) -> (w763:bool, error out=w764:errorcluster)
            n213 = case shown="True" w763 {
              tunnel: w764 -> [w768 w773]
              tunnel: [w770 w774] -> w766
              frame False {
                w769 = FALSE ("K1")
                n214 = shared-variable "RT CompactRIO Target\\SCADALib.lvlib\\K1"(w769, error in=w768) -> (error out=w767:errorcluster)
                n215 = shared-variable "RT CompactRIO Target\\Mod8\\DO2"(w769, error in=w767) -> (error out=w770:errorcluster)
              }
              frame True {
                n216 = shared-variable "RT CompactRIO Target\\Mod7\\DI7"(error in=w773) -> (w772:bool, error out=w771:errorcluster)
                n217 = case shown="True" w772 {
                  tunnel: w771 -> [w776 w780]
                  tunnel: [w778 w782] -> w774
                  frame False {
                    w777 = TRUE ("K1")
                    n218 = shared-variable "RT CompactRIO Target\\SCADALib.lvlib\\K1"(w777, error in=w776) -> (error out=w775:errorcluster)
                    n219 = shared-variable "RT CompactRIO Target\\Mod8\\DO2"(w777, error in=w775) -> (error out=w778:errorcluster)
                  }
                  frame True {
                    w781 = FALSE ("K1")
                    n220 = shared-variable "RT CompactRIO Target\\SCADALib.lvlib\\K1"(w781, error in=w780) -> (error out=w779:errorcluster)
                    n221 = shared-variable "RT CompactRIO Target\\Mod8\\DO2"(w781, error in=w779) -> (error out=w782:errorcluster)
                  }
                }
              }
            }
          }
        }
        n222 = shared-variable "RT CompactRIO Target\\Mod7\\DI2"(error in=w622) -> (w612:bool, error out=w609:errorcluster)
        n223 = shared-variable "RT CompactRIO Target\\SCADALib.lvlib\\Emergency Stop"(error in=w609) -> (w610:bool, error out=w605:errorcluster)
        n224 = And(x=w610, y=w612) -> (x .and. y?=w611:bool)
        n225 = shared-variable "RT CompactRIO Target\\SCADALib.lvlib\\Stop"(error in=w605) -> (w606:bool, error out=w604:errorcluster)
        n226 = shared-variable "RT CompactRIO Target\\Mod7\\DI1"(error in=w604) -> (w608:bool, error out=w613:errorcluster)
        n227 = And(x=w606, y=w608) -> (x .and. y?=w607:bool)
        n228 = Select(t=w630, s=w611, f=T2."Emergency Shutdown" ("Stanja")) -> (s? t:f=w633:T2)
        n229 = case shown="True" w607 {
          tunnel: [TRUE w638] -> w618
          tunnel: [w635 w637] -> w614
          tunnel: w613 -> [w635 w637]
          frame False {
          }
          frame True {
            n230 = local read "Stop"() -> (w638:bool)
          }
        }
        n231 = Merge Errors(w614, w632) -> (w631:errorcluster)
        n232 = Not(x=w611) -> (.not. x?=w616:bool)
      }
      frame "K6" {
        w786 = T2."Emergency Shutdown" ("Stanja")
        w785 = FALSE ("DO2")
        n233 = shared-variable "RT CompactRIO Target\\Mod8\\DO2"(w785, error in=w800) -> (error out=w784:errorcluster)
        n234 = shared-variable "RT CompactRIO Target\\SCADALib.lvlib\\K1"(w785, error in=w784) -> (error out=w783:errorcluster)
        n235 = shared-variable "RT CompactRIO Target\\Mod7\\DI7"(error in=w783) -> (w804:bool, error out=w805:errorcluster)
        n236 = case shown="False" w804 {
          tunnel: [w815 T2."K6" ("Stanja")] -> w806
          tunnel: w805 -> [w813 w827]
          tunnel: [w814 w829] -> w798
          frame False {
            n237 = shared-variable "RT CompactRIO Target\\Mod7\\DI11"(error in=w813) -> (w812:bool, error out=w811:errorcluster)
            n238 = case shown="False" w812 {
              tunnel: [T2."K6" ("Stanja") T2."Sledeci paket" ("Stanja")] -> w815
              tunnel: w811 -> [w817 w822]
              tunnel: [w819 w824] -> w814
              frame False {
                w818 = TRUE ("K6")
                n239 = shared-variable "RT CompactRIO Target\\SCADALib.lvlib\\K6"(w818, error in=w817) -> (error out=w816:errorcluster)
                n240 = shared-variable "RT CompactRIO Target\\Mod8\\DO7"(w818, error in=w816) -> (error out=w819:errorcluster)
              }
              frame True {
                w823 = FALSE ("K6")
                n241 = shared-variable "RT CompactRIO Target\\SCADALib.lvlib\\K6"(w823, error in=w822) -> (error out=w821:errorcluster)
                n242 = shared-variable "RT CompactRIO Target\\Mod8\\DO7"(w823, error in=w821) -> (error out=w824:errorcluster)
              }
            }
          }
          frame True {
            w828 = FALSE ("K6")
            n243 = shared-variable "RT CompactRIO Target\\SCADALib.lvlib\\K6"(w828, error in=w827) -> (error out=w826:errorcluster)
            n244 = shared-variable "RT CompactRIO Target\\Mod8\\DO7"(w828, error in=w826) -> (error out=w829:errorcluster)
          }
        }
        n245 = shared-variable "RT CompactRIO Target\\Mod7\\DI1"(error in=w798) -> (w797:bool, error out=w794:errorcluster)
        n246 = shared-variable "RT CompactRIO Target\\SCADALib.lvlib\\Stop"(error in=w794) -> (w795:bool, error out=w793:errorcluster)
        n247 = And(x=w795, y=w797) -> (x .and. y?=w796:bool)
        n248 = case shown="False" w796 {
          tunnel: [TRUE w810] -> w803
          tunnel: w793 -> [w807 w809]
          tunnel: [w807 w809] -> w799
          frame False {
          }
          frame True {
            n249 = local read "Stop"() -> (w810:bool)
          }
        }
        n250 = shared-variable "RT CompactRIO Target\\Mod7\\DI2"(error in=w799) -> (w790:bool, error out=w792:errorcluster)
        n251 = shared-variable "RT CompactRIO Target\\SCADALib.lvlib\\Emergency Stop"(error in=w792) -> (w789:bool, error out=w791:errorcluster)
        n252 = Select(t=w806, s=w790, f=w786) -> (s? t:f=w787:T2)
        n253 = Select(t=w787, s=w789, f=w786) -> (s? t:f=w788:T2)
        n254 = Not(x=w790) -> (.not. x?=w802:bool)
      }
      frame "K5" {
        n255 = shared-variable "RT CompactRIO Target\\Mod7\\DI3"(error in=w851) -> (w855:bool, error out=w841:errorcluster)
        n256 = shared-variable "RT CompactRIO Target\\Mod8\\DO6"(TRUE ("K5"), error in=w851) -> (error out=w850:errorcluster)
        n257 = shared-variable "RT CompactRIO Target\\Mod8\\DO8"(FALSE ("K7"), error in=w850) -> (error out=w852:errorcluster)
        n258 = shared-variable "RT CompactRIO Target\\Mod8\\DO7"(FALSE ("K6"), error in=w852) -> (error out=w837:errorcluster)
        n259 = case shown="True" w855 {
          tunnel: w841 -> [w866 w872]
          tunnel: [w865 w876] -> w858
          frame False {
            n260 = shared-variable "RT CompactRIO Target\\Mod8\\DO2"(TRUE ("K1"), error in=w866) -> (error out=w865:errorcluster)
          }
          frame True {
            n261 = shared-variable "RT CompactRIO Target\\Mod7\\DI11"(error in=w872) -> (w871:bool, error out=w869:errorcluster)
            n262 = shared-variable "RT CompactRIO Target\\Mod7\\DI11"(error in=w869) -> (w870:bool, error out=w868:errorcluster)
            n263 = xnode "Edge Detect"("error in"=w868, "input 1"=w870) -> ("error out"=w875:errorcluster, "output"=w874:bool)  [unwired: 1 in]
            n264 = Or(x=w874, y=w871) -> (x .or. y?=w873:bool)
            n265 = case shown="True" w873 {
              tunnel: w875 -> [w918 w922]
              tunnel: [w917 w923] -> w876
              frame False {
                n266 = shared-variable "RT CompactRIO Target\\Mod8\\DO2"(FALSE ("K1"), error in=w918) -> (error out=w917:errorcluster)
              }
              frame True {
                n267 = shared-variable "RT CompactRIO Target\\Mod7\\DI7"(error in=w922) -> (w920:bool, error out=w921:errorcluster)
                n268 = case shown="False" w920 {
                  tunnel: w921 -> [w925 w928]
                  tunnel: [w924 w927] -> w923
                  frame False {
                    n269 = shared-variable "RT CompactRIO Target\\Mod8\\DO2"(TRUE ("K1"), error in=w925) -> (error out=w924:errorcluster)
                  }
                  frame True {
                    n270 = shared-variable "RT CompactRIO Target\\Mod8\\DO2"(FALSE ("K1"), error in=w928) -> (error out=w927:errorcluster)
                  }
                }
              }
            }
          }
        }
        n271 = case shown="False" w855 {
          tunnel: [T2."K5" ("Stanja") w935] -> w856
          tunnel: [w930 w933] -> w833
          tunnel: w841 -> [w930 w932]
          frame True {
          }
          frame False {
            n272 = local read "Trenutni paket"() -> (w934:enum16{"Nema paketa", "P1", "P2", "P3"})
            n273 = case shown="\"P1\", Default" w934 {
              tunnel: [T2."K2" ("Stanja") T2."K7" ("Stanja") T2."K7" ("Stanja")] -> w935
              tunnel: [w936 w938 w940] -> w933
              tunnel: w932 -> [w936 w938 w940]
              frame "P1", Default {
              }
              frame "P2" {
              }
              frame "P3" {
              }
            }
          }
        }
        n274 = shared-variable "RT CompactRIO Target\\SCADALib.lvlib\\Emergency Stop"(error in=w833) -> (w834:bool, error out=w832:errorcluster)
        n275 = shared-variable "RT CompactRIO Target\\Mod7\\DI2"(error in=w832) -> (w831:bool, error out=w848:errorcluster)
        n276 = shared-variable "RT CompactRIO Target\\SCADALib.lvlib\\Stop"(error in=w837) -> (w838:bool, error out=w836:errorcluster)
        n277 = shared-variable "RT CompactRIO Target\\Mod7\\DI1"(error in=w836) -> (w839:bool, error out=w843:errorcluster)
        n278 = And(x=w838, y=w839) -> (x .and. y?=w840:bool)
        n279 = And(x=w834, y=w831) -> (x .and. y?=w835:bool)
        n280 = case shown="True" w840 {
          tunnel: [TRUE w864] -> w847
          tunnel: w843 -> [w861 w863]
          tunnel: [w861 w863] -> w842
          frame False {
          }
          frame True {
            n281 = local read "Stop"() -> (w864:bool)
          }
        }
        n282 = Merge Errors(w842, w858) -> (w857:errorcluster)
        n283 = Select(t=w856, s=w835, f=T2."Emergency Shutdown" ("Stanja")) -> (s? t:f=w859:T2)
        n284 = Not(x=w835) -> (.not. x?=w845:bool)
        n285 = Merge Errors(w857, w848) -> (w860:errorcluster)
      }
      frame "K3" {
        w943 = TRUE ("K5")
        w942 = FALSE ("K7")
        n286 = shared-variable "RT CompactRIO Target\\Mod8\\DO4"(w943, error in=w965) -> (error out=w964:errorcluster)
        n287 = shared-variable "RT CompactRIO Target\\Mod8\\DO6"(w943, error in=w964) -> (error out=w966:errorcluster)
        n288 = shared-variable "RT CompactRIO Target\\SCADALib.lvlib\\K5"(w943) -> ()  [unwired: 1 in, 1 out]
        n289 = shared-variable "RT CompactRIO Target\\SCADALib.lvlib\\K3"(w943) -> ()  [unwired: 1 in, 1 out]
        n290 = shared-variable "RT CompactRIO Target\\Mod8\\DO8"(w942, error in=w966) -> (error out=w963:errorcluster)
        n291 = shared-variable "RT CompactRIO Target\\Mod7\\DI9"(error in=w963) -> (w962:bool, error out=w955:errorcluster)
        n292 = shared-variable "RT CompactRIO Target\\SCADALib.lvlib\\K7"(w942) -> ()  [unwired: 1 in, 1 out]
        n293 = shared-variable "RT CompactRIO Target\\SCADALib.lvlib\\K1"(w942) -> ()  [unwired: 1 in, 1 out]
        n294 = shared-variable "RT CompactRIO Target\\Mod8\\DO2"(w942, error in=w955) -> (error out=w954:errorcluster)
        n295 = case shown="False" w962 {
          tunnel: [T2."K6" ("Stanja") T2."K3" ("Stanja")] -> w967
          tunnel: [w973 w975] -> w945
          tunnel: w954 -> [w973 w975]
          frame True {
          }
          frame False {
          }
        }
        n296 = shared-variable "RT CompactRIO Target\\SCADALib.lvlib\\Emergency Stop"(error in=w945) -> (w946:bool, error out=w944:errorcluster)
        n297 = shared-variable "RT CompactRIO Target\\Mod7\\DI2"(error in=w944) -> (w947:bool, error out=w950:errorcluster)
        n298 = And(x=w947, y=w946) -> (x .and. y?=w948:bool)
        n299 = shared-variable "RT CompactRIO Target\\SCADALib.lvlib\\Stop"(error in=w950) -> (w951:bool, error out=w949:errorcluster)
        n300 = Select(t=w967, s=w948, f=T2."Emergency Shutdown") -> (s? t:f=w968:T2)
        n301 = shared-variable "RT CompactRIO Target\\Mod7\\DI1"(error in=w949) -> (w953:bool, error out=w956:errorcluster)
        n302 = Not(x=w948) -> (.not. x?=w959:bool)
        n303 = And(x=w951, y=w953) -> (x .and. y?=w952:bool)
        n304 = case shown="False" w952 {
          tunnel: [TRUE w972] -> w961
          tunnel: [w969 w971] -> w957
          tunnel: w956 -> [w969 w971]
          frame False {
          }
          frame True {
            n305 = local read "Stop"() -> (w972:bool)
          }
        }
      }
      frame "K4" {
        w977 = TRUE ("K5")
        w978 = FALSE ("K7")
        n306 = shared-variable "RT CompactRIO Target\\Mod8\\DO5"(w977, error in=w1000) -> (error out=w999:errorcluster)
        n307 = shared-variable "RT CompactRIO Target\\Mod8\\DO6"(w977, error in=w999) -> (error out=w1001:errorcluster)
        n308 = shared-variable "RT CompactRIO Target\\SCADALib.lvlib\\K3"(w977) -> ()  [unwired: 1 in, 1 out]
        n309 = shared-variable "RT CompactRIO Target\\Mod8\\DO8"(w978, error in=w1001) -> (error out=w998:errorcluster)
        n310 = shared-variable "RT CompactRIO Target\\Mod7\\DI10"(error in=w998) -> (w997:bool, error out=w992:errorcluster)
        n311 = shared-variable "RT CompactRIO Target\\SCADALib.lvlib\\K5"(w977) -> ()  [unwired: 1 in, 1 out]
        n312 = shared-variable "RT CompactRIO Target\\SCADALib.lvlib\\K7"(w978) -> ()  [unwired: 1 in, 1 out]
        n313 = shared-variable "RT CompactRIO Target\\Mod8\\DO2"(w978, error in=w992) -> (error out=w991:errorcluster)
        n314 = shared-variable "RT CompactRIO Target\\SCADALib.lvlib\\K1"(w978) -> ()  [unwired: 1 in, 1 out]
        n315 = case shown="True" w997 {
          tunnel: [T2."K6" ("Stanja") T2."K4" ("Stanja")] -> w1002
          tunnel: [w1008 w1010] -> w980
          tunnel: w991 -> [w1008 w1010]
          frame True {
          }
          frame False {
          }
        }
        n316 = shared-variable "RT CompactRIO Target\\SCADALib.lvlib\\Emergency Stop"(error in=w980) -> (w981:bool, error out=w979:errorcluster)
        n317 = shared-variable "RT CompactRIO Target\\Mod7\\DI2"(error in=w979) -> (w982:bool, error out=w985:errorcluster)
        n318 = And(x=w982, y=w981) -> (x .and. y?=w983:bool)
        n319 = shared-variable "RT CompactRIO Target\\SCADALib.lvlib\\Stop"(error in=w985) -> (w986:bool, error out=w984:errorcluster)
        n320 = shared-variable "RT CompactRIO Target\\Mod7\\DI1"(error in=w984) -> (w988:bool, error out=w989:errorcluster)
        n321 = Select(t=w1002, s=w983, f=T2."Emergency Shutdown") -> (s? t:f=w1003:T2)
        n322 = Not(x=w983) -> (.not. x?=w994:bool)
        n323 = And(x=w986, y=w988) -> (x .and. y?=w987:bool)
        n324 = case shown="True" w987 {
          tunnel: [TRUE w1007] -> w996
          tunnel: [w1004 w1006] -> w990
          tunnel: w989 -> [w1004 w1006]
          frame False {
          }
          frame True {
            n325 = local read "Stop"() -> (w1007:bool)
          }
        }
      }
      frame "K2" {
        w1012 = TRUE ("K2")
        n326 = shared-variable "RT CompactRIO Target\\Mod7\\DI8"(error in=w1023) -> (w1036:bool, error out=w1024:errorcluster)
        n327 = shared-variable "RT CompactRIO Target\\SCADALib.lvlib\\K2"(w1012) -> ()  [unwired: 1 in, 1 out]
        n328 = shared-variable "RT CompactRIO Target\\Mod8\\DO3"(w1012, error in=w1023) -> (error out=w1031:errorcluster)
        n329 = shared-variable "RT CompactRIO Target\\Mod7\\DI3"(error in=w1031) -> (w1033:bool, error out=w1032:errorcluster)
        n330 = case shown="False" w1036 {
          tunnel: [T2."Sledeci paket" ("Stanja") T2."K2" ("Stanja")] -> w1037
          tunnel: w1024 -> [w1049 w1051]
          tunnel: [w1048 w1051] -> w1014
          frame True {
            w1047 = TRUE ("K1")
            n331 = shared-variable "RT CompactRIO Target\\SCADALib.lvlib\\K1"(w1047) -> ()  [unwired: 1 in, 1 out]
            n332 = shared-variable "RT CompactRIO Target\\Mod8\\DO2"(w1047, error in=w1049) -> (error out=w1048:errorcluster)
          }
          frame False {
          }
        }
        n333 = case shown="False" w1033 {
          tunnel: [w1043 w1046] -> w1019
          tunnel: w1032 -> [w1043 w1045]
          frame False {
          }
          frame True {
            w1044 = FALSE ("K1")
            n334 = shared-variable "RT CompactRIO Target\\Mod8\\DO2"(w1044, error in=w1045) -> (error out=w1046:errorcluster)
            n335 = shared-variable "RT CompactRIO Target\\SCADALib.lvlib\\K1"(w1044) -> ()  [unwired: 1 in, 1 out]
          }
        }
        n336 = shared-variable "RT CompactRIO Target\\SCADALib.lvlib\\Emergency Stop"(error in=w1014) -> (w1015:bool, error out=w1013:errorcluster)
        n337 = shared-variable "RT CompactRIO Target\\SCADALib.lvlib\\Stop"(error in=w1019) -> (w1020:bool, error out=w1018:errorcluster)
        n338 = shared-variable "RT CompactRIO Target\\Mod7\\DI2"(error in=w1013) -> (w1016:bool, error out=w1035:errorcluster)
        n339 = shared-variable "RT CompactRIO Target\\Mod7\\DI1"(error in=w1018) -> (w1022:bool, error out=w1025:errorcluster)
        n340 = And(x=w1015, y=w1016) -> (x .and. y?=w1017:bool)
        n341 = And(x=w1020, y=w1022) -> (x .and. y?=w1021:bool)
        n342 = Select(t=w1037, s=w1017, f=T2."Emergency Shutdown") -> (s? t:f=w1038:T2)
        n343 = case shown="True" w1021 {
          tunnel: [TRUE w1042] -> w1030
          tunnel: [w1039 w1041] -> w1026
          tunnel: w1025 -> [w1039 w1041]
          frame False {
          }
          frame True {
            n344 = local read "Stop"() -> (w1042:bool)
          }
        }
        n345 = Not(x=w1017) -> (.not. x?=w1028:bool)
        n346 = Merge Errors(w1026, w1035) -> (w1034:errorcluster)
      }
      frame "Emergency Shutdown" {
        n347 = local read "Emergency Stop"() -> (w1071:bool)
        n348 = case shown="True" w1071 {
          selector: w1071 -> [w1162 _]
          tunnel: w1054 -> [w1163 w1188]
          tunnel: [w1163 w1169] -> w1060
          tunnel: [w1162 w1168] -> w1058
          frame False {
          }
          frame True {
            w1168 = FALSE
            n349 = shared-variable "RT CompactRIO Target\\Mod8\\DO0"(error in=w1188) -> (→"DO0":bool, error out=w1187:errorcluster)
            n350 = shared-variable "RT CompactRIO Target\\Mod8\\DO1"(error in=w1187) -> (→"DO1":bool, error out=w1186:errorcluster)
            n351 = shared-variable "RT CompactRIO Target\\Mod8\\DO2"(error in=w1186) -> (→"DO2":bool, error out=w1185:errorcluster)
            n352 = shared-variable "RT CompactRIO Target\\Mod8\\DO3"(error in=w1185) -> (→"DO3":bool, error out=w1184:errorcluster)
            n353 = shared-variable "RT CompactRIO Target\\Mod8\\DO4"(error in=w1184) -> (→"DO4":bool, error out=w1183:errorcluster)
            n354 = shared-variable "RT CompactRIO Target\\Mod8\\DO5"(error in=w1183) -> (→"DO5":bool, error out=w1182:errorcluster)
            n355 = shared-variable "RT CompactRIO Target\\Mod8\\DO6"(error in=w1182) -> (→"DO6":bool, error out=w1181:errorcluster)
            n356 = shared-variable "RT CompactRIO Target\\Mod8\\DO7"(error in=w1181) -> (→"DO7":bool, error out=w1180:errorcluster)
            n357 = shared-variable "RT CompactRIO Target\\Mod8\\DO8"(error in=w1180) -> (→"DO8":bool, error out=w1179:errorcluster)
            n358 = shared-variable "RT CompactRIO Target\\Mod8\\DO9"(error in=w1179) -> (→"DO9":bool, error out=w1178:errorcluster)
            n359 = shared-variable "RT CompactRIO Target\\Mod8\\DO10"(error in=w1178) -> (→"DO10":bool, error out=w1177:errorcluster)
            n360 = shared-variable "RT CompactRIO Target\\Mod8\\DO11"(error in=w1177) -> (→"DO11":bool, error out=w1176:errorcluster)
            n361 = shared-variable "RT CompactRIO Target\\Mod8\\DO12"(error in=w1176) -> (→"DO12":bool, error out=w1175:errorcluster)
            n362 = local read "Timer Data Out za drugi sprat"() -> (w1196:T3)
            n363 = local read "Timer Data Out za treci sprat"() -> (w1197:T3)
            n364 = local read "Timer Data Out za prvi sprat"() -> (w1206:T3)
            n365 = local read "Stanja tajmera za sprat 3"() -> (→"Stanja tajmera 3 - sacuvano":enum16{"Running", "Waiting"})
            n366 = local read "Stanja tajmera za sprat 1"() -> (→"Stanje tajmera 1 - sacuvano":enum16{"Running", "Waiting"})
            n367 = local read "Stanja tajmera za sprat 2"() -> (→"Stanja tajmera 2 - sacuvano":enum16{"Running", "Waiting"})
            n368 = Unbundle By Name(w1206) -> ("Elapsed Time"=w1205:dbl)
            n369 = Unbundle By Name(w1196) -> ("Elapsed Time"=w1200:dbl)
            n370 = Unbundle By Name(w1197) -> ("Elapsed Time"=w1199:dbl)
            n371 = shared-variable "RT CompactRIO Target\\Mod8\\DO13"(error in=w1175) -> (→"DO13":bool, error out=w1174:errorcluster)
            n372 = shared-variable "RT CompactRIO Target\\Mod8\\DO14"(error in=w1174) -> (→"DO14":bool, error out=w1173:errorcluster)
            n373 = shared-variable "RT CompactRIO Target\\Mod8\\DO15"(error in=w1173) -> (→"DO15":bool, error out=w1172:errorcluster)
            n374 = local write "Emergency Stop"(w1168) -> ()
            n375 = Subtract(x=30.0, y=w1205) -> (x-y=→"Vreme 1":dbl)
            n376 = Subtract(x=30.0, y=w1200) -> (x-y=→"Vreme 2":dbl)
            n377 = Subtract(x=30.0, y=w1199) -> (x-y=→"Vreme 3":dbl)
            n378 = call "Nastajmer.vi"("error in (no error)"=w1172, "Enum"=Control_Timer."Reset") -> ("error out"=w1171:errorcluster)  [unwired: 7 in, 2 out]
            n379 = call "Nastajmer2.vi"("error in (no error)"=w1171, "Enum"=Control_Timer2."Reset") -> ("error out"=w1170:errorcluster)  [unwired: 7 in, 2 out]
            n380 = call "Nastajmer3.vi"("error in (no error)"=w1170, "Enum"=Control_Timer3."Reset") -> ("error out"=w1169:errorcluster)  [unwired: 7 in, 2 out]
          }
        }
        n381 = shared-variable "RT CompactRIO Target\\SCADALib.lvlib\\Emergency Stop"(error in=w1054) -> (w1055:bool, error out=w1053:errorcluster)
        n382 = shared-variable "RT CompactRIO Target\\Mod7\\DI2"(error in=w1053) -> (w1057:bool, error out=w1068:errorcluster)
        n383 = And(x=w1055, y=w1057) -> (x .and. y?=w1056:bool)
        n384 = Not(x=w1071) -> (.not. x?=w1070:bool)
        n385 = And(x=w1070, y=w1056) -> (x .and. y?=w1069:bool)
        n386 = case shown="True" w1069 {
          tunnel: [T2."Emergency Shutdown" ("Stanja") w1100] -> w1073
          tunnel: w1068 -> [w1088 w1094]
          tunnel: [w1077 w1098] -> w1067
          frame False {
            w1075 = TRUE
            w1076 = FALSE
            n387 = shared-variable "RT CompactRIO Target\\SCADALib.lvlib\\K7"(w1076) -> ()  [unwired: 1 in, 1 out]
            n388 = shared-variable "RT CompactRIO Target\\SCADALib.lvlib\\K4"(w1076) -> ()  [unwired: 1 in, 1 out]
            n389 = shared-variable "RT CompactRIO Target\\SCADALib.lvlib\\K2"(w1076) -> ()  [unwired: 1 in, 1 out]
            n390 = shared-variable "RT CompactRIO Target\\SCADALib.lvlib\\K3"(w1076) -> ()  [unwired: 1 in, 1 out]
            n391 = shared-variable "RT CompactRIO Target\\SCADALib.lvlib\\K1"(w1076) -> ()  [unwired: 1 in, 1 out]
            n392 = shared-variable "RT CompactRIO Target\\SCADALib.lvlib\\K5"(w1076) -> ()  [unwired: 1 in, 1 out]
            n393 = shared-variable "RT CompactRIO Target\\SCADALib.lvlib\\K6"(w1076) -> ()  [unwired: 1 in, 1 out]
            n394 = shared-variable "RT CompactRIO Target\\SCADALib.lvlib\\On-Off"(w1076) -> ()  [unwired: 1 in, 1 out]
            n395 = shared-variable "RT CompactRIO Target\\Mod8\\DO0"(w1076, error in=w1088) -> (error out=w1087:errorcluster)
            n396 = shared-variable "RT CompactRIO Target\\Mod8\\DO2"(w1076, error in=w1087) -> (error out=w1086:errorcluster)
            n397 = shared-variable "RT CompactRIO Target\\Mod8\\DO3"(w1076, error in=w1086) -> (error out=w1085:errorcluster)
            n398 = shared-variable "RT CompactRIO Target\\Mod8\\DO4"(w1076, error in=w1085) -> (error out=w1084:errorcluster)
            n399 = shared-variable "RT CompactRIO Target\\Mod8\\DO5"(w1076, error in=w1084) -> (error out=w1083:errorcluster)
            n400 = shared-variable "RT CompactRIO Target\\Mod8\\DO6"(w1076, error in=w1083) -> (error out=w1082:errorcluster)
            n401 = shared-variable "RT CompactRIO Target\\Mod8\\DO7"(w1076, error in=w1082) -> (error out=w1081:errorcluster)
            n402 = shared-variable "RT CompactRIO Target\\Mod8\\DO8"(w1076, error in=w1081) -> (error out=w1080:errorcluster)
            n403 = shared-variable "RT CompactRIO Target\\SCADALib.lvlib\\H9"(w1075) -> ()  [unwired: 1 in, 1 out]
            n404 = shared-variable "RT CompactRIO Target\\Mod8\\DO15"(w1075, error in=w1080) -> (error out=w1079:errorcluster)
            n405 = shared-variable "RT CompactRIO Target\\Mod8\\DO1"(w1075, error in=w1079) -> (error out=w1078:errorcluster)
            n406 = shared-variable "RT CompactRIO Target\\SCADALib.lvlib\\Fault"(w1075, error in=w1078) -> (error out=w1077:errorcluster)
            n407 = local write "Stanja tajmera za sprat 1"(enum16{"Running", "Waiting"}."Waiting" ("Stanja tajmera za spratove 1")) -> ()
            n408 = local write "Stanja tajmera za sprat 3"(enum16{"Running", "Waiting"}."Waiting" ("Stanja tajmera za spratove 1")) -> ()
            n409 = local write "Stanja tajmera za sprat 2"(enum16{"Running", "Waiting"}."Waiting" ("Stanja tajmera za spratove 1")) -> ()
          }
          frame True {
            n410 = shared-variable "RT CompactRIO Target\\SCADALib.lvlib\\Start"(error in=w1094) -> (w1095:bool, error out=w1093:errorcluster)
            n411 = shared-variable "RT CompactRIO Target\\Mod7\\DI0"(error in=w1093) -> (w1096:bool, error out=w1099:errorcluster)
            n412 = Exclusive Or(1:w1095, 2:w1096) -> (0:w1097:bool)
            n413 = case shown="True" w1097 {
              tunnel: [T2."Emergency Shutdown" ("Stanja") w1161] -> w1100
              tunnel: w1099 -> [w1101 w1122]
              tunnel: [w1101 w1103] -> w1098
              frame False {
              }
              frame True {
                w1124 = FALSE
                n414 = local read "DO8"() -> (w1132:bool)
                n415 = local read "DO6"() -> (w1134:bool)
                n416 = local read "DO2"() -> (w1137:bool)
                n417 = local read "DO7"() -> (w1133:bool)
                n418 = local read "DO0"() -> (w1140:bool)
                n419 = local read "DO3"() -> (w1136:bool)
                n420 = local read "DO1"() -> (w1138:bool)
                n421 = local read "DO4"() -> (w1135:bool)
                n422 = local read "DO5"() -> (w1123:bool)
                n423 = shared-variable "RT CompactRIO Target\\SCADALib.lvlib\\K1"(w1137, error in=w1122) -> (error out=w1121:errorcluster)
                n424 = shared-variable "RT CompactRIO Target\\SCADALib.lvlib\\Fault"(w1138, error in=w1121) -> (error out=w1120:errorcluster)
                n425 = shared-variable "RT CompactRIO Target\\SCADALib.lvlib\\On-Off"(w1140, error in=w1120) -> (error out=w1119:errorcluster)
                n426 = shared-variable "RT CompactRIO Target\\SCADALib.lvlib\\K2"(w1136, error in=w1119) -> (error out=w1118:errorcluster)
                n427 = shared-variable "RT CompactRIO Target\\SCADALib.lvlib\\K3"(w1135, error in=w1118) -> (error out=w1117:errorcluster)
                n428 = shared-variable "RT CompactRIO Target\\SCADALib.lvlib\\K4"(w1123, error in=w1117) -> (error out=w1116:errorcluster)
                n429 = shared-variable "RT CompactRIO Target\\SCADALib.lvlib\\K5"(w1134, error in=w1116) -> (error out=w1115:errorcluster)
                n430 = shared-variable "RT CompactRIO Target\\SCADALib.lvlib\\K6"(w1133, error in=w1115) -> (error out=w1114:errorcluster)
                n431 = shared-variable "RT CompactRIO Target\\SCADALib.lvlib\\K7"(w1132, error in=w1114) -> (error out=w1113:errorcluster)
                n432 = local read "Stanja tajmera 2 - sacuvano"() -> (w1159:enum16{"Running", "Waiting"})
                n433 = local read "Stanje tajmera 1 - sacuvano"() -> (w1160:enum16{"Running", "Waiting"})
                n434 = local read "Stanja tajmera 3 - sacuvano"() -> (w1158:enum16{"Running", "Waiting"})
                n435 = shared-variable "RT CompactRIO Target\\Mod8\\DO0"(w1140, error in=w1122) -> (error out=w1157:errorcluster)
                n436 = shared-variable "RT CompactRIO Target\\Mod8\\DO1"(w1138, error in=w1157) -> (error out=w1156:errorcluster)
                n437 = shared-variable "RT CompactRIO Target\\Mod8\\DO2"(w1137, error in=w1156) -> (error out=w1155:errorcluster)
                n438 = shared-variable "RT CompactRIO Target\\Mod8\\DO3"(w1136, error in=w1155) -> (error out=w1154:errorcluster)
                n439 = shared-variable "RT CompactRIO Target\\Mod8\\DO4"(w1135, error in=w1154) -> (error out=w1153:errorcluster)
                n440 = shared-variable "RT CompactRIO Target\\Mod8\\DO5"(w1123, error in=w1153) -> (error out=w1152:errorcluster)
                n441 = shared-variable "RT CompactRIO Target\\Mod8\\DO6"(w1134, error in=w1152) -> (error out=w1151:errorcluster)
                n442 = shared-variable "RT CompactRIO Target\\Mod8\\DO7"(w1133, error in=w1151) -> (error out=w1150:errorcluster)
                n443 = shared-variable "RT CompactRIO Target\\Mod8\\DO8"(w1132, error in=w1150) -> (error out=w1149:errorcluster)
                n444 = local read "DO14"() -> (w1126:bool)
                n445 = local read "DO15"() -> (w1125:bool)
                n446 = local read "DO10"() -> (w1131:bool)
                n447 = local read "DO9"() -> (w1130:bool)
                n448 = local read "DO13"() -> (w1127:bool)
                n449 = local read "DO11"() -> (w1129:bool)
                n450 = local read "DO12"() -> (w1128:bool)
                n451 = shared-variable "RT CompactRIO Target\\SCADALib.lvlib\\H3"(w1130, error in=w1113) -> (error out=w1112:errorcluster)
                n452 = shared-variable "RT CompactRIO Target\\SCADALib.lvlib\\H4"(w1131, error in=w1112) -> (error out=w1111:errorcluster)
                n453 = local write "Stanja tajmera za sprat 2"(w1159) -> ()
                n454 = local write "Stanja tajmera za sprat 1"(w1160) -> ()
                n455 = shared-variable "RT CompactRIO Target\\SCADALib.lvlib\\H5"(w1129, error in=w1111) -> (error out=w1110:errorcluster)
                n456 = shared-variable "RT CompactRIO Target\\SCADALib.lvlib\\H6"(w1128, error in=w1110) -> (error out=w1109:errorcluster)
                n457 = shared-variable "RT CompactRIO Target\\SCADALib.lvlib\\H7"(w1127, error in=w1109) -> (error out=w1108:errorcluster)
                n458 = shared-variable "RT CompactRIO Target\\SCADALib.lvlib\\H8"(w1126, error in=w1108) -> (error out=w1107:errorcluster)
                n459 = shared-variable "RT CompactRIO Target\\SCADALib.lvlib\\H9"(w1125, error in=w1107) -> (error out=w1106:errorcluster)
                n460 = local write "Stanja tajmera za sprat 3"(w1158) -> ()
                n461 = local read "Sacuvano stanje"() -> (w1161:T2)
                n462 = shared-variable "RT CompactRIO Target\\Mod8\\DO9"(w1130, error in=w1149) -> (error out=w1148:errorcluster)
                n463 = shared-variable "RT CompactRIO Target\\Mod8\\DO10"(w1131, error in=w1148) -> (error out=w1147:errorcluster)
                n464 = shared-variable "RT CompactRIO Target\\Mod8\\DO11"(w1129, error in=w1147) -> (error out=w1146:errorcluster)
                n465 = shared-variable "RT CompactRIO Target\\Mod8\\DO12"(w1128, error in=w1146) -> (error out=w1145:errorcluster)
                n466 = shared-variable "RT CompactRIO Target\\Mod8\\DO13"(w1127, error in=w1145) -> (error out=w1144:errorcluster)
                n467 = shared-variable "RT CompactRIO Target\\Mod8\\DO14"(w1126, error in=w1144) -> (error out=w1143:errorcluster)
                n468 = shared-variable "RT CompactRIO Target\\Mod8\\DO15"(w1125, error in=w1143) -> (error out=w1142:errorcluster)
                n469 = shared-variable "RT CompactRIO Target\\SCADALib.lvlib\\H9"(w1124, error in=w1106) -> (error out=w1104:errorcluster)
                n470 = shared-variable "RT CompactRIO Target\\Mod8\\DO15"(w1124, error in=w1142) -> (error out=w1141:errorcluster)
                n471 = shared-variable "RT CompactRIO Target\\Mod8\\DO1"(w1124, error in=w1141) -> (error out=w1139:errorcluster)
                n472 = shared-variable "RT CompactRIO Target\\SCADALib.lvlib\\Fault"(w1124, error in=w1139) -> (error out=w1105:errorcluster)
                n473 = Merge Errors(w1105, w1104) -> (w1103:errorcluster)
              }
            }
          }
        }
        n474 = shared-variable "RT CompactRIO Target\\SCADALib.lvlib\\Stop"(error in=w1060) -> (w1061:bool, error out=w1059:errorcluster)
        n475 = shared-variable "RT CompactRIO Target\\Mod7\\DI1"(error in=w1059) -> (w1063:bool, error out=w1064:errorcluster)
        n476 = And(x=w1061, y=w1063) -> (x .and. y?=w1062:bool)
        n477 = case shown="False" w1062 {
          tunnel: [TRUE w1222] -> w1074
          tunnel: [w1219 w1221] -> w1065
          tunnel: w1064 -> [w1219 w1221]
          frame False {
          }
          frame True {
            n478 = local read "Stop"() -> (w1222:bool)
          }
        }
        n479 = local read "Sacuvano stanje"() -> (w1072:T2)
        n480 = Merge Errors(w1065, w1067) -> (w1066:errorcluster)
      }
      frame "Shutdown" {
        n481 = shared-variable "RT CompactRIO Target\\SCADALib.lvlib\\Stop"(error in=w1224) -> (w1226:bool, error out=w1223:errorcluster)
        n482 = shared-variable "RT CompactRIO Target\\Mod7\\DI1"(error in=w1223) -> (w1227:bool, error out=w1228:errorcluster)
        n483 = And(x=w1226, y=w1227) -> (x .and. y?=w1225:bool)
        n484 = case shown="True" w1225 {
          tunnel: [TRUE w1237] -> w1232
          tunnel: [w1234 w1236] -> w1229
          tunnel: w1228 -> [w1234 w1236]
          frame False {
          }
          frame True {
            n485 = local read "Stop"() -> (w1237:bool)
          }
        }
      }
      frame "P1" {
        w1240 = TRUE ("DO2")
        n486 = shared-variable "RT CompactRIO Target\\Mod7\\DI11"(error in=w1261) -> (w1259:bool, error out=w1260:errorcluster)
        n487 = shared-variable "RT CompactRIO Target\\Mod7\\DI3"(error in=w1260) -> (w1262:bool, error out=w1239:errorcluster)
        n488 = shared-variable "RT CompactRIO Target\\SCADALib.lvlib\\K1"(w1240, error in=w1239) -> (error out=w1238:errorcluster)
        n489 = shared-variable "RT CompactRIO Target\\Mod8\\DO2"(w1240, error in=w1238) -> (error out=w1247:errorcluster)
        n490 = And(x=w1262, y=w1259) -> (x .and. y?=w1265:bool)
        n491 = case shown="False" w1265 {
          tunnel: [T2."P1" ("Stanja") T2."K5" ("Stanja")] -> w1263
          tunnel: [w1270 w1272] -> w1242
          tunnel: w1239 -> [w1270 w1274]
          frame False {
          }
          frame True {
            w1275 = TRUE
            n492 = shared-variable "RT CompactRIO Target\\SCADALib.lvlib\\K5"(w1275, error in=w1274) -> (error out=w1273:errorcluster)
            n493 = shared-variable "RT CompactRIO Target\\Mod8\\DO6"(w1275, error in=w1273) -> (error out=w1272:errorcluster)
          }
        }
        n494 = shared-variable "RT CompactRIO Target\\SCADALib.lvlib\\Emergency Stop"(error in=w1242) -> (w1243:bool, error out=w1241:errorcluster)
        n495 = shared-variable "RT CompactRIO Target\\Mod7\\DI2"(error in=w1241) -> (w1244:bool, error out=w1254:errorcluster)
        n496 = shared-variable "RT CompactRIO Target\\SCADALib.lvlib\\Stop"(error in=w1247) -> (w1248:bool, error out=w1246:errorcluster)
        n497 = And(x=w1243, y=w1244) -> (x .and. y?=w1245:bool)
        n498 = shared-variable "RT CompactRIO Target\\Mod7\\DI1"(error in=w1246) -> (w1250:bool, error out=w1251:errorcluster)
        n499 = Select(t=w1263, s=w1245, f=T2."Emergency Shutdown") -> (s? t:f=w1264:T2)
        n500 = And(x=w1248, y=w1250) -> (x .and. y?=w1249:bool)
        n501 = case shown="True" w1249 {
          tunnel: [TRUE w1269] -> w1258
          tunnel: [w1266 w1268] -> w1252
          tunnel: w1251 -> [w1266 w1268]
          frame False {
          }
          frame True {
            n502 = local read "Stop"() -> (w1269:bool)
          }
        }
        n503 = Not(x=w1245) -> (.not. x?=w1256:bool)
        n504 = Merge Errors(w1252, w1254) -> (w1253:errorcluster)
      }
      frame "P2" {
        w1279 = TRUE ("DO2")
        n505 = shared-variable "RT CompactRIO Target\\Mod7\\DI11"(error in=w1300) -> (w1298:bool, error out=w1299:errorcluster)
        n506 = shared-variable "RT CompactRIO Target\\Mod7\\DI3"(error in=w1299) -> (w1301:bool, error out=w1278:errorcluster)
        n507 = And(x=w1301, y=w1298) -> (x .and. y?=w1304:bool)
        n508 = shared-variable "RT CompactRIO Target\\SCADALib.lvlib\\K1"(w1279, error in=w1278) -> (error out=w1277:errorcluster)
        n509 = shared-variable "RT CompactRIO Target\\Mod8\\DO2"(w1279, error in=w1277) -> (error out=w1287:errorcluster)
        n510 = case shown="False" w1304 {
          tunnel: [T2."P2" ("Stanja") T2."K5" ("Stanja")] -> w1302
          tunnel: w1278 -> [w1309 w1314]
          tunnel: [w1309 w1311] -> w1281
          frame False {
          }
          frame True {
            w1313 = TRUE
            n511 = shared-variable "RT CompactRIO Target\\Mod8\\DO6"(w1313, error in=w1314) -> (error out=w1312:errorcluster)
            n512 = shared-variable "RT CompactRIO Target\\SCADALib.lvlib\\K5"(w1313, error in=w1312) -> (error out=w1311:errorcluster)
          }
        }
        n513 = shared-variable "RT CompactRIO Target\\SCADALib.lvlib\\Emergency Stop"(error in=w1281) -> (w1282:bool, error out=w1280:errorcluster)
        n514 = shared-variable "RT CompactRIO Target\\Mod7\\DI2"(error in=w1280) -> (w1283:bool, error out=w1293:errorcluster)
        n515 = shared-variable "RT CompactRIO Target\\SCADALib.lvlib\\Stop"(error in=w1287) -> (w1285:bool, error out=w1286:errorcluster)
        n516 = shared-variable "RT CompactRIO Target\\Mod7\\DI1"(error in=w1286) -> (w1289:bool, error out=w1290:errorcluster)
        n517 = And(x=w1282, y=w1283) -> (x .and. y?=w1284:bool)
        n518 = Select(t=w1302, s=w1284, f=T2."Emergency Shutdown") -> (s? t:f=w1303:T2)
        n519 = And(x=w1285, y=w1289) -> (x .and. y?=w1288:bool)
        n520 = case shown="True" w1288 {
          tunnel: [TRUE w1308] -> w1297
          tunnel: [w1305 w1307] -> w1291
          tunnel: w1290 -> [w1305 w1307]
          frame False {
          }
          frame True {
            n521 = local read "Stop"() -> (w1308:bool)
          }
        }
        n522 = Merge Errors(w1291, w1293) -> (w1292:errorcluster)
        n523 = Not(x=w1284) -> (.not. x?=w1294:bool)
      }
      frame "P3" {
        w1318 = TRUE ("DO2")
        n524 = shared-variable "RT CompactRIO Target\\Mod7\\DI11"(error in=w1339) -> (w1337:bool, error out=w1338:errorcluster)
        n525 = shared-variable "RT CompactRIO Target\\Mod7\\DI3"(error in=w1338) -> (w1340:bool, error out=w1317:errorcluster)
        n526 = And(x=w1340, y=w1337) -> (x .and. y?=w1343:bool)
        n527 = shared-variable "RT CompactRIO Target\\SCADALib.lvlib\\K1"(w1318, error in=w1317) -> (error out=w1316:errorcluster)
        n528 = shared-variable "RT CompactRIO Target\\Mod8\\DO2"(w1318, error in=w1316) -> (error out=w1325:errorcluster)
        n529 = case shown="True" w1343 {
          tunnel: [T2."P3" ("Stanja") T2."K5" ("Stanja")] -> w1341
          tunnel: [w1348 w1353] -> w1320
          tunnel: w1317 -> [w1348 w1351]
          frame False {
          }
          frame True {
            w1352 = TRUE
            n530 = shared-variable "RT CompactRIO Target\\SCADALib.lvlib\\K5"(w1352, error in=w1351) -> (error out=w1350:errorcluster)
            n531 = shared-variable "RT CompactRIO Target\\Mod8\\DO6"(w1352, error in=w1350) -> (error out=w1353:errorcluster)
          }
        }
        n532 = shared-variable "RT CompactRIO Target\\SCADALib.lvlib\\Emergency Stop"(error in=w1320) -> (w1321:bool, error out=w1319:errorcluster)
        n533 = shared-variable "RT CompactRIO Target\\SCADALib.lvlib\\Stop"(error in=w1325) -> (w1326:bool, error out=w1324:errorcluster)
        n534 = shared-variable "RT CompactRIO Target\\Mod7\\DI2"(error in=w1319) -> (w1322:bool, error out=w1332:errorcluster)
        n535 = shared-variable "RT CompactRIO Target\\Mod7\\DI1"(error in=w1324) -> (w1328:bool, error out=w1329:errorcluster)
        n536 = And(x=w1321, y=w1322) -> (x .and. y?=w1323:bool)
        n537 = And(x=w1326, y=w1328) -> (x .and. y?=w1327:bool)
        n538 = Select(t=w1341, s=w1323, f=T2."Emergency Shutdown") -> (s? t:f=w1342:T2)
        n539 = case shown="True" w1327 {
          tunnel: [TRUE w1347] -> w1336
          tunnel: [w1344 w1346] -> w1330
          tunnel: w1329 -> [w1344 w1346]
          frame False {
          }
          frame True {
            n540 = local read "Stop"() -> (w1347:bool)
          }
        }
        n541 = Not(x=w1323) -> (.not. x?=w1334:bool)
        n542 = Merge Errors(w1330, w1332) -> (w1331:errorcluster)
      }
    }
    "Stop" <- w386
    "Emergency Stop" <- w385
    "Sacuvano stanje" <- w384
    n543 = shared-variable "RT CompactRIO Target\\SCADALib.lvlib\\S1"(w379, error in=w362) -> (error out=w361:errorcluster)
    n544 = shared-variable "RT CompactRIO Target\\SCADALib.lvlib\\S2"(w378, error in=w361) -> (error out=w360:errorcluster)
    n545 = shared-variable "RT CompactRIO Target\\SCADALib.lvlib\\S3"(w377, error in=w360) -> (error out=w359:errorcluster)
    n546 = shared-variable "RT CompactRIO Target\\Mod7\\DI3"(error in=w359) -> (w376:bool, error out=w358:errorcluster)
    n547 = shared-variable "RT CompactRIO Target\\Mod7\\DI4"(error in=w358) -> (w375:bool, error out=w357:errorcluster)
    n548 = shared-variable "RT CompactRIO Target\\Mod7\\DI5"(error in=w357) -> (w374:bool, error out=w356:errorcluster)
    n549 = shared-variable "RT CompactRIO Target\\SCADALib.lvlib\\B1"(w376, error in=w356) -> (error out=w355:errorcluster)
    n550 = shared-variable "RT CompactRIO Target\\SCADALib.lvlib\\B2"(w375, error in=w355) -> (error out=w354:errorcluster)
    n551 = shared-variable "RT CompactRIO Target\\SCADALib.lvlib\\B3"(w374, error in=w354) -> (error out=w353:errorcluster)
    n552 = shared-variable "RT CompactRIO Target\\Mod7\\DI6"(error in=w353) -> (w373:bool, error out=w352:errorcluster)
    n553 = shared-variable "RT CompactRIO Target\\Mod7\\DI7"(error in=w352) -> (w372:bool, error out=w351:errorcluster)
    n554 = shared-variable "RT CompactRIO Target\\Mod7\\DI8"(error in=w351) -> (w371:bool, error out=w350:errorcluster)
    n555 = shared-variable "RT CompactRIO Target\\SCADALib.lvlib\\B4"(w373, error in=w350) -> (error out=w349:errorcluster)
    n556 = shared-variable "RT CompactRIO Target\\SCADALib.lvlib\\B5"(w372, error in=w349) -> (error out=w348:errorcluster)
    n557 = shared-variable "RT CompactRIO Target\\SCADALib.lvlib\\B6"(w371, error in=w348) -> (error out=w347:errorcluster)
    n558 = shared-variable "RT CompactRIO Target\\Mod7\\DI9"(error in=w347) -> (w370:bool, error out=w346:errorcluster)
    n559 = shared-variable "RT CompactRIO Target\\Mod7\\DI10"(error in=w346) -> (w369:bool, error out=w345:errorcluster)
    n560 = shared-variable "RT CompactRIO Target\\Mod7\\DI11"(error in=w345) -> (w368:bool, error out=w344:errorcluster)
    n561 = shared-variable "RT CompactRIO Target\\Mod7\\DI12"(error in=w344) -> (w367:bool, error out=w343:errorcluster)
    n562 = shared-variable "RT CompactRIO Target\\Mod7\\DI13"(error in=w343) -> (w366:bool, error out=w342:errorcluster)
    n563 = shared-variable "RT CompactRIO Target\\SCADALib.lvlib\\B7"(w370, error in=w342) -> (error out=w341:errorcluster)
    n564 = shared-variable "RT CompactRIO Target\\SCADALib.lvlib\\B8"(w369, error in=w341) -> (error out=w340:errorcluster)
    n565 = shared-variable "RT CompactRIO Target\\SCADALib.lvlib\\B9"(w368, error in=w340) -> (error out=w339:errorcluster)
    n566 = shared-variable "RT CompactRIO Target\\SCADALib.lvlib\\B10"(w367, error in=w339) -> (error out=w338:errorcluster)
    n567 = shared-variable "RT CompactRIO Target\\SCADALib.lvlib\\B11"(w366, error in=w338) -> (error out=w337:errorcluster)
    n568 = case shown="\"Wait\", Default" w383 {
      tunnel: w337 -> [w398 w411]
      tunnel: [w389 w405] -> w382
      frame "Wait", Default {
        n569 = shared-variable "RT CompactRIO Target\\Mod7\\DI8"(error in=w398) -> (w399:bool, error out=w397:errorcluster)
        n570 = shared-variable "RT CompactRIO Target\\Mod7\\DI9"(error in=w397) -> (w402:bool, error out=w396:errorcluster)
        n571 = shared-variable "RT CompactRIO Target\\Mod7\\DI10"(error in=w396) -> (w404:bool, error out=w395:errorcluster)
        n572 = shared-variable "RT CompactRIO Target\\Mod8\\DO9"(w399, error in=w395) -> (error out=w394:errorcluster)
        n573 = shared-variable "RT CompactRIO Target\\Mod8\\DO11"(w402, error in=w394) -> (error out=w393:errorcluster)
        n574 = shared-variable "RT CompactRIO Target\\Mod8\\DO13"(w404, error in=w393) -> (error out=w392:errorcluster)
        n575 = Not(x=w404) -> (.not. x?=w403:bool)
        n576 = Not(x=w399) -> (.not. x?=w400:bool)
        n577 = Not(x=w402) -> (.not. x?=w401:bool)
        n578 = shared-variable "RT CompactRIO Target\\Mod8\\DO10"(w400, error in=w392) -> (error out=w391:errorcluster)
        n579 = shared-variable "RT CompactRIO Target\\Mod8\\DO12"(w401, error in=w391) -> (error out=w390:errorcluster)
        n580 = shared-variable "RT CompactRIO Target\\Mod8\\DO14"(w403, error in=w390) -> (error out=w389:errorcluster)
      }
      frame "Emergency Shutdown" {
        w412 = TRUE
        n581 = shared-variable "RT CompactRIO Target\\Mod8\\DO9"(w412, error in=w411) -> (error out=w410:errorcluster)
        n582 = shared-variable "RT CompactRIO Target\\Mod8\\DO11"(w412, error in=w410) -> (error out=w409:errorcluster)
        n583 = shared-variable "RT CompactRIO Target\\Mod8\\DO13"(w412, error in=w409) -> (error out=w408:errorcluster)
        n584 = Not(x=w412) -> (.not. x?=w415:bool)
        n585 = Not(x=w412) -> (.not. x?=w413:bool)
        n586 = Not(x=w412) -> (.not. x?=w414:bool)
        n587 = shared-variable "RT CompactRIO Target\\Mod8\\DO10"(w413, error in=w408) -> (error out=w407:errorcluster)
        n588 = shared-variable "RT CompactRIO Target\\Mod8\\DO12"(w414, error in=w407) -> (error out=w406:errorcluster)
        n589 = shared-variable "RT CompactRIO Target\\Mod8\\DO14"(w415, error in=w406) -> (error out=w405:errorcluster)
      }
    }
    n590 = Merge Errors(w381, w382) -> (w380:errorcluster)
    "Trenutno stanje" <- w383
  }
  n591 = local write "Trenutni paket"(w18) -> ()
  n592 = local write "Sledeci paket"(w18) -> ()
  n593 = while {
    shift-right: [w1361] -> w8
    shift-left: "error in" -> [w1357]
    stop <- FALSE stop-if-true
    n594 = shared-variable "RT CompactRIO Target\\Mod7\\DI4"(error in=w1357) -> (w1358:bool, error out=w1356:errorcluster)
    n595 = xnode "Edge Detect"("error in"=w1356, "input 1"=w1358) -> ("error out"=w1359:errorcluster, "output"=w1360:bool)  [unwired: 1 in]
    n596 = case shown="False" w1360 {
      tunnel: [w1404 w1409] -> w1361
      tunnel: w1359 -> [w1404 w1407]
      tunnel: [w1403 w1408] -> w1355
      frame False {
        n597 = local read "Sledeci paket"() -> (w1403:enum16{"Nema paketa", "P1", "P2", "P3"})
      }
      frame True {
        n598 = shared-variable "RT CompactRIO Target\\Mod7\\DI6"(error in=w1407) -> (w1405:bool, error out=w1406:errorcluster)
        n599 = case shown="False" w1405 {
          tunnel: [w1410 w1416] -> w1409
          tunnel: [enum16{"Nema paketa", "P1", "P2", "P3"}."P2" ("Paketi") w1415] -> w1408
          tunnel: w1406 -> [w1410 w1412]
          frame False {
          }
          frame True {
            n600 = shared-variable "RT CompactRIO Target\\Mod7\\DI5"(error in=w1412) -> (w1414:bool, error out=w1413:errorcluster)
            n601 = case shown="False" w1414 {
              tunnel: w1413 -> [w1418 w1420]
              tunnel: [w1418 w1420] -> w1416
              tunnel: [enum16{"Nema paketa", "P1", "P2", "P3"}."P1" ("Paketi") enum16{"Nema paketa", "P1", "P2", "P3"}."P3" ("Paketi")] -> w1415
              frame False {
              }
              frame True {
              }
            }
          }
        }
      }
    }
    "Sledeci paket" <- w1355
  }
  n602 = Merge Errors(w8, w7, w1) -> (→"error out":errorcluster)
